vi "index.vi"() -> ()   [LabVIEW 2026]
uses:
  <vilib>/Utility/miscctls.llb/LVPoint32TypeDef.ctl
  <vilib>/Utility/miscctls.llb/LVRectTypeDef.ctl
  <vilib>/Utility/miscctls.llb/LVPointTypeDef.ctl
  <vilib>/Instr/_visa.llb/VISA Flush IO Buffer Mask.ctl
  <userlib>/Sensor.ctl
  <vilib>/measure/maspectr.llb/FFT Spectrum (Mag-Phase) for N Chan.vi
  <vilib>/Analysis/3filter.llb/Butterworth Filter (DBL).vi
  <vilib>/Instr/_visa.llb/VISA Configure Serial Port (Instr).vi
  <vilib>/measure/NI_MAPro.lvlib
  <vilib>/Analysis/NI_AALBase.lvlib
panel:
  out "AlphaxBeta":bool
  out "CoordsEEGBeta":T1 {"Čas (s)" format="%#.2f"; "Amplituda (mV)" format="%#.3f"}
  out "CoordsEEGAlpha":T1 {"Čas (s)" format="%#.2f"; "Amplituda (mV)" format="%#.3f"}
  out "SyncStopEEG":bool
  out "SyncStopACC":bool
  out "CoordsACC":T1 {"Čas (s)" format="%#.2f"; "Amplituda (mV)" format="%#.3f"}
  out "CoordsEMG":T1 {"Čas (s)" format="%#.2f"; "Amplituda (mV)" format="%#.3f"}
  out "EKGxHRV":bool
  out "CoordsHRV":T1 {"Čas (s)" format="%#.2f"; "Amplituda (mV)" format="%#.3f"}
  out "CoordsEKG":T1 {"Čas (s)" format="%#.2f"; "Amplituda (mV)" format="%#.3f"}
  out "GraphEEG2":waveform(dbl)(graph)
  out "GraphEEG1":waveform(dbl)(graph)
  out "error out 7":errorcluster
  out "error out 6":errorcluster
  out "RawEEG":waveform(dbl)(graph)
  out "size(s) 3":i32
  out "size(s) 4":i32
  out "error out 5":errorcluster
  out "error out 4":errorcluster
  out "Vzorkovacka 2":dbl
  out "RawACC":waveform(dbl)
  out "vzorkovackaEEG":dbl
  out "RawEMG":waveform(dbl)
  out "error out 3":errorcluster
  out "error out 2":errorcluster
  out "error out":errorcluster
  out "RawEKG":waveform(dbl)
  out "array":dbl[](array[numeric])
  out "Vzorkovacka":dbl
  out "SyncStopEMG":bool
  in  "Time Target (s)":dbl=60.0
  out "SyncStopEKG":bool
  in  "UvodniStranka":bool
  in  "ExitApp":bool
  in  "error in (no error)":errorcluster
  in  "Tab Control":T2(tab)
  in  "Playground":bool
  in  "UlohaACC":bool
  in  "UlohaEEG":bool
  in  "UlohaEMG":bool
  in  "UlohaEKG":bool
  out "EKGHRV":cluster{dbl[], dbl[]}(graph)
  in  "Délka časového okna (s)":dbl=1.0 min=1.0 max=20.0 step=1.0
  in  "Zobrazit graf č.":dbl min=0.0 max=0.0 step=1.0
  in  "DeleteSignalEKG":bool
  in  "StartMeasureEKG":bool
  in  "HintEKG":bool
  out "GraphEKG":waveform(dbl)[](graph)
  out "ChartEKG":dbl(graph)
  in  "Vstupní COM port 2":refnum<visa-resource-name>
  out "BPM":i32
  in  "Doba měření (s)":dbl=1.0 caption="Time Target (s)"
  in  "SaveCSV":bool
  in  "SavePNG":bool
  out "InfoCursor":cluster{"Čas (s)":dbl, "Amplituda (mV)":dbl}[](array[cluster]) {"Amplituda (mV)" format="%#.2f"; "Čas (s)" format="%#.2f"}
  in  "StopMeasureEKG":bool
  out "InfoCursorEEG":cluster{"Čas (s)":dbl, "Amplituda (mV)":dbl}[](array[cluster]) {"Amplituda (mV)" format="%#.2f"; "Čas (s)" format="%#.2f"}
  in  "Časové okno všech signálů (s)":dbl min=0.0 max=20.0 step=1.0
  in  "Zobrazit signál č._EEG":dbl min=0.0 max=1.0
  in  "HintEEG":bool
  in  "DeleteSignalEEG":bool
  in  "StartMeasureEEG":bool
  in  "Doba měření (s)":dbl
  in  "Vstupní COM port 4":refnum<visa-resource-name>
  out "GraphEEG4":waveform(dbl)(graph)
  out "GraphEEG3":waveform(dbl)(graph)
  out "ChartEEG":dbl(graph)
  in  "SaveCSVEEG":bool
  in  "StopMeasureEEG":bool
  out "InfoCursorACC":cluster{"Čas (s)":dbl, "Amplituda (mV)":dbl}[](array[cluster]) {"Amplituda (mV)" format="%#.2f"; "Čas (s)" format="%#.2f"}
  in  "SaveCSVACC":bool
  in  "SavePNGACC":bool
  in  "Délka časového okna (s) ACC":dbl=1.0 min=1.0 max=20.0 step=1.0
  in  "Zobrazit signál č._ACC":dbl min=0.0 max=1.0
  in  "HintACC":bool
  out "GraphACC":waveform(dbl)[](graph)
  out "ChartACC":dbl(graph)
  in  "DeleteSignalACC":bool
  in  "StartMeasureACC":bool
  in  "Doba měření (s) ACC":dbl
  in  "Vstupní COM port ACC":refnum<visa-resource-name>
  in  "StopMeasureACC":bool
  out "InfoCursorEMG":cluster{"Čas (s)":dbl, "Amplituda (mV)":dbl}[](array[cluster]) {"Amplituda (mV)" format="%#.2f"; "Čas (s)" format="%#.2f"}
  in  "SaveCSVEMG":bool
  in  "SavePNGEMG":bool
  in  "Délka časového okna (s) EMG":dbl=1.0 min=1.0 max=20.0 step=1.0
  in  "Zobrazit signál č.":dbl min=0.0 max=2.0
  in  "HintEMG":bool
  out "GraphEMG":waveform(dbl)[](graph)
  out "ChartEMG":dbl(graph)
  in  "DeleteSignalEMG":bool
  in  "StartMeasureEMG":bool
  in  "Doba měření (s)":dbl
  in  "Vstupní COM port 3":refnum<visa-resource-name>
  in  "StopMeasureEMG":bool
  out "SpectrumPlayground":cluster{"f0":dbl, "df":dbl, "magnitude":dbl[]}[](graph)
  in  "Filtr":bool
  in  "SaveFileButton":bool
  out "Waveform Graph":waveform(dbl)[](graph)
  in  "Horní mezní frekvence":dbl=0.45000000000000007 format="%0.2f"
  in  "Dolní mezní frekvence":dbl=0.12500000000000006 format="%0.4f"
  in  "Typ filtru":T3(ring)
  in  "OdstranitFiltr":bool
  in  "Cluster":T4
  in  "DeleteSignal":bool
  out "Waveform Chart":dbl[](graph)
  in  "SendToFilter":bool
  out "Waveform":waveform(dbl)[](graph)
  out "SyncStop":bool
  in  "Vstupní COM port":refnum<visa-resource-name>
  in  "Vzorkovací frekvence (Hz)":enum16{"1", "10", "100", "1000"}(ring)
  in  "Druh signálu":T5
  in  "StartMeasure":bool
  in  "StopMeasure":bool
  in  "index":i32
  # "CHYBÍ UDĚLAT SMARTKURSOR A STOP BUTTON U EEG\nUDĚLAT VŠECHNY PROTOKOLY\nUDĚLAT PEAK COUNTER V AKCELEROMETRU\nFIXNOUT VOLNÉ MĚŘENÍ"
  # "Aplikace pro měření na platformě PLUX BITalino"
  # "Úloha č. 1 - měření a vyhodnocení EKG signálu"
  # "Vstupní COM port"
  # "Kurzor"
  # "Amplituda (mV) / BPM (-)"
  # "Čas (s)"
  # "Úloha č. 3 - měření a vyhodnocení EEG signálu"
  # "Vstupní COM port"
  # "Zobrazit graf č."
  # "Alfa"
  # "Beta"
  # "Kurzor"
  # "Amplituda (uV)"
  # "Čas (s)"
  # "EDA"
  # "Úloha č. 4 - měření a vyhodnocení signálu Z - akcelerometru"
  # "Vstupní COM port"
  # "Doba měření (s)"
  # "Zobrazit signál č."
  # "Délka časového okna (s)"
  # "Kurzor"
  # "Amplituda (g)"
  # "Čas (s)"
  # "Úloha č. 2 - měření a vyhodnocení EMG signálu"
  # "Vstupní COM port"
  # "Délka časového okna (s)"
  # "Kurzor"
  # "Amplituda (mV)"
  # "Čas (s)"
  # "A1"
  # "A2"
  # "A3"
  # "A4"
  # "A5"
  # "A6"
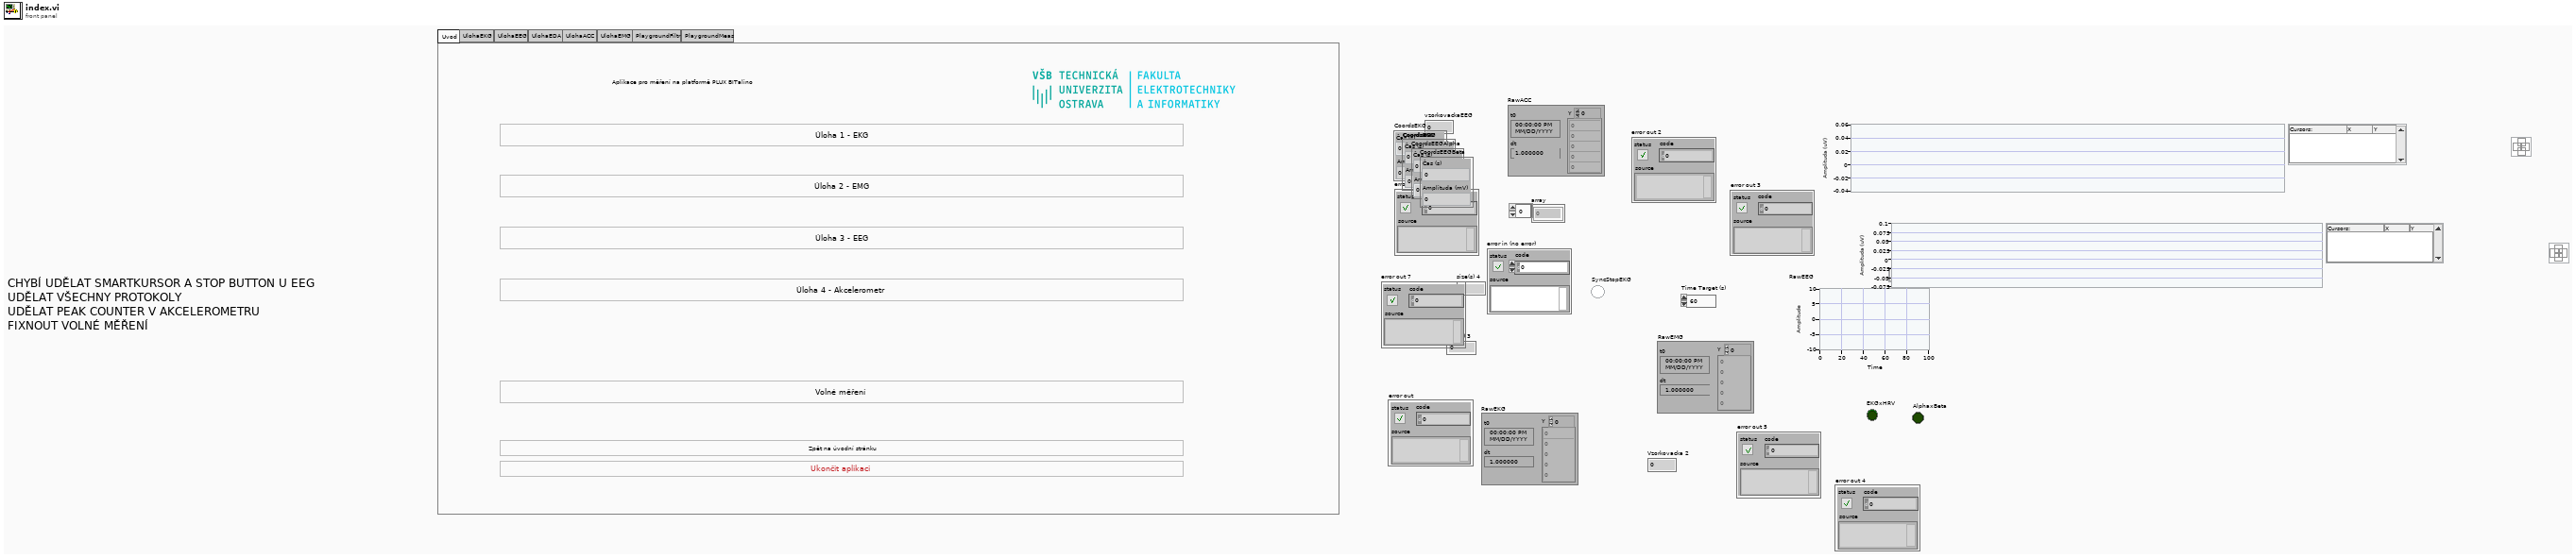
[diagram p1: front panel]
types:
  T1 = typedef "LVPoint32TypeDef.ctl" = cluster{"Čas (s)":dbl, "Amplituda (mV)":dbl}
  T2 = enum32{"Uvod", "UlohaEKG", "UlohaEEG", "UlohaEDA", "UlohaACC", "UlohaEMG", "PlaygroundFiltr", "PlaygroundMeas"}
  T3 = enum32{"Lowpass", "Highpass", "Bandpass", "Bandstop"}
  T4 = cluster{"A1":bool, "A2":bool, "A3":bool, "A4":bool, "A5":bool, "A6":bool}
  T5 = cluster{"Signál na kanálu A1":enum16{"EMG", "ECG", "EEG", "EDA", "ACC"}, "Signál na kanálu A2":enum16{"EMG", "ECG", "EEG", "EDA", "ACC"}, "Signál na kanálu A3":enum16{"EMG", "ECG", "EEG", "EDA", "ACC"}, "Signál na kanálu A4":enum16{"EMG", "ECG", "EEG", "EDA", "ACC"}, "Signál na kanálu A5":enum16{"EMG", "ECG", "EEG", "EDA", "ACC"}, "Signál na kanálu A6":enum16{"EMG", "ECG", "EEG", "EDA", "ACC"}}
  T6 = enum16{"Always On", "Always Off", "Off While Running"}
  T7 = enum16{"Wait", "Exit", "Measure", "Intro", "UlohaEKG", "UlohaEMG", "PlaygroundMeas", "UlohaEEG", "UlohaEDA", "UlohaACC", "PlaygroundFiltr", "SaveFile", "FilterSignal", "RemoveFilter", "HintEKG", "DeleteSignal", "DeleteSignalEKG", "HintEMG", "HintEEG", "DeleteSignalEMG", "StartMeasureEEG", "DeleteSignalEEG", "ShowGraphECG", "ChangeTimeECG", "SavePNG", "SaveCSV", "ChangeTimeEMG", "ShowGraphEMG", "ShowGraphEEG", "ShowGraphACC", "ChangeTimeACC", "DeleteSignalACC", "HintACC", "ChangeTimeEEG", "Cursor"}
  T8 = enum32{"Uvod", "UlohaEKG", "UlohaEEG", "UlohaEDA", "UlohaACC", "UlohaEMG", "PlaygroundFiltr"}
  T9 = typedef "LVPointTypeDef.ctl" = cluster{"Horizontal":i16, "Vertical":i16}
  T10 = typedef "LVRectTypeDef.ctl" = cluster{"Left":i16, "Top":i16, "Right":i16, "Bottom":i16}
  T11 = enum8{"Enabled", "Disabled", "Disabled and Grayed Out"}
  T12 = typedef "Sensor.ctl" = enum16{"EMG", "ECG", "EEG", "EDA", "ACC", "LUX"}
  T13 = cluster{"Sensor 1":T12, "Sensor 2":T12, "Sensor 3":T12, "Sensor 4":T12, "Sensor 5":T12, "Sensor 6":T12}
  T14 = typedef "VISA Flush IO Buffer Mask.ctl" = u16
  T15 = cluster{"Result":dbl, "Result":dbl, "Result":dbl, "Result":dbl, "Result":dbl, "Result":dbl}
  T16 = enum16{"Wait", "Exit", "Measure", "Intro", "UlohaEKG", "UlohaEMG", "PlaygroundMeas", "UlohaEEG", "UlohaEDA", "UlohaACC", "PlaygroundFiltr", "SaveFile", "FilterSignal", "RemoveFilter", "HintEKG"}
  T17 = enum16{"Wait", "Exit", "Measure", "Intro", "UlohaEKG", "UlohaEMG", "PlaygroundMeas", "UlohaEEG", "UlohaEDA", "UlohaACC"}
  T18 = enum16{"Wait", "Exit", "Measure", "Intro", "UlohaEKG", "UlohaEMG", "PlaygroundMeas"}
  T19 = enum16{"Wait", "Exit", "Measure", "Intro", "UlohaEKG", "UlohaEMG"}
  T20 = enum16{"Wait", "Exit", "Measure", "Intro", "UlohaEKG", "UlohaEMG", "PlaygroundMeas", "UlohaEEG", "UlohaEDA", "UlohaACC", "PlaygroundFiltr", "SaveFile", "FilterSignal", "RemoveFilter", "HintEKG", "DeleteSignal", "DeleteSignalEKG", "HintEMG", "HintEEG", "DeleteSignalEMG", "StartMeasureEEG", "DeleteSignalEEG", "ShowGraphECG", "ChangeTimeECG", "SavePNG", "SaveCSV", "ChangeTimeEMG", "ShowGraphEMG", "ShowGraphEEG", "ShowGraphACC", "ChangeTimeACC", "DeleteSignalACC"}
  T21 = enum16{"Wait", "Exit", "Measure", "Intro", "UlohaEKG", "UlohaEMG", "PlaygroundMeas", "UlohaEEG", "UlohaEDA", "UlohaACC", "PlaygroundFiltr", "SaveFile", "FilterSignal", "RemoveFilter", "HintEKG", "DeleteSignal"}
  T22 = enum16{"Wait", "Exit", "Measure", "Intro", "UlohaEKG", "UlohaEMG", "PlaygroundMeas", "UlohaEEG", "UlohaEDA", "UlohaACC", "PlaygroundFiltr", "SaveFile", "FilterSignal", "RemoveFilter", "HintEKG", "DeleteSignal", "DeleteSignalEKG"}
  T23 = enum16{"Wait", "Exit", "Measure", "Intro", "UlohaEKG", "UlohaEMG", "PlaygroundMeas", "UlohaEEG", "UlohaEDA", "UlohaACC", "PlaygroundFiltr", "SaveFile", "FilterSignal", "RemoveFilter", "HintEKG", "DeleteSignal", "DeleteSignalEKG", "HintEMG", "HintEEG", "DeleteSignalEMG"}
  T24 = enum16{"Wait", "Exit", "Measure", "Intro", "UlohaEKG", "UlohaEMG", "PlaygroundMeas", "UlohaEEG", "UlohaEDA", "UlohaACC", "PlaygroundFiltr", "SaveFile", "FilterSignal", "RemoveFilter", "HintEKG", "DeleteSignal", "DeleteSignalEKG", "HintEMG", "HintEEG", "DeleteSignalEMG", "StartMeasureEEG", "DeleteSignalEEG"}
  T25 = enum16{"Wait", "Exit", "Measure", "Intro", "UlohaEKG", "UlohaEMG", "PlaygroundMeas", "UlohaEEG", "UlohaEDA", "UlohaACC", "PlaygroundFiltr", "SaveFile", "FilterSignal", "RemoveFilter", "HintEKG", "DeleteSignal", "DeleteSignalEKG", "HintEMG", "HintEEG", "DeleteSignalEMG", "StartMeasureEEG", "DeleteSignalEEG", "ShowGraphECG", "ChangeTimeECG"}
  T26 = enum16{"Wait", "Exit", "Measure", "Intro", "UlohaEKG", "UlohaEMG", "PlaygroundMeas", "UlohaEEG", "UlohaEDA", "UlohaACC", "PlaygroundFiltr", "SaveFile", "FilterSignal", "RemoveFilter", "HintEKG", "DeleteSignal", "DeleteSignalEKG", "HintEMG", "HintEEG", "DeleteSignalEMG", "StartMeasureEEG", "DeleteSignalEEG", "ShowGraphECG", "ChangeTimeECG", "SavePNG", "SaveCSV", "ChangeTimeEMG"}
  T27 = enum16{"Wait", "Exit", "Measure", "Intro", "UlohaEKG", "UlohaEMG", "PlaygroundMeas", "UlohaEEG", "UlohaEDA", "UlohaACC", "PlaygroundFiltr", "SaveFile", "FilterSignal", "RemoveFilter", "HintEKG", "DeleteSignal", "DeleteSignalEKG", "HintEMG", "HintEEG", "DeleteSignalEMG", "StartMeasureEEG", "DeleteSignalEEG", "ShowGraphECG", "ChangeTimeECG", "SavePNG", "SaveCSV", "ChangeTimeEMG", "ShowGraphEMG", "ShowGraphEEG", "ShowGraphACC", "ChangeTimeACC", "DeleteSignalACC", "HintACC", "ChangeTimeEEG"}
  T28 = enum16{"Wait", "Exit", "Measure", "Intro", "UlohaEKG", "UlohaEMG", "PlaygroundMeas", "UlohaEEG", "UlohaEDA", "UlohaACC", "PlaygroundFiltr", "SaveFile", "FilterSignal", "RemoveFilter", "HintEKG", "DeleteSignal", "DeleteSignalEKG", "HintEMG", "HintEEG", "DeleteSignalEMG", "StartMeasureEEG", "DeleteSignalEEG", "ShowGraphECG", "ChangeTimeECG", "SavePNG"}
  T29 = enum16{"Wait", "Exit", "Measure", "Intro", "UlohaEKG", "UlohaEMG", "PlaygroundMeas", "UlohaEEG", "UlohaEDA", "UlohaACC", "PlaygroundFiltr", "SaveFile", "FilterSignal", "RemoveFilter", "HintEKG", "DeleteSignal", "DeleteSignalEKG", "HintEMG", "HintEEG", "DeleteSignalEMG", "StartMeasureEEG", "DeleteSignalEEG", "ShowGraphECG", "ChangeTimeECG", "SavePNG", "SaveCSV"}
  T30 = enum16{"Wait", "Exit", "Measure", "Intro", "UlohaEKG", "UlohaEMG", "PlaygroundMeas", "UlohaEEG", "UlohaEDA", "UlohaACC", "PlaygroundFiltr", "SaveFile", "FilterSignal", "RemoveFilter", "HintEKG", "DeleteSignal", "DeleteSignalEKG", "HintEMG", "HintEEG", "DeleteSignalEMG", "StartMeasureEEG", "DeleteSignalEEG", "ShowGraphECG", "ChangeTimeECG", "SavePNG", "SaveCSV", "ChangeTimeEMG", "ShowGraphEMG", "ShowGraphEEG"}
  T31 = enum16{"Wait", "Exit", "Measure", "Intro", "UlohaEKG", "UlohaEMG", "PlaygroundMeas", "UlohaEEG", "UlohaEDA", "UlohaACC", "PlaygroundFiltr", "SaveFile", "FilterSignal", "RemoveFilter", "HintEKG", "DeleteSignal", "DeleteSignalEKG", "HintEMG", "HintEEG", "DeleteSignalEMG", "StartMeasureEEG", "DeleteSignalEEG", "ShowGraphECG", "ChangeTimeECG", "SavePNG", "SaveCSV", "ChangeTimeEMG", "ShowGraphEMG"}
  T32 = enum16{"Wait", "Exit", "Measure", "Intro", "UlohaEKG", "UlohaEMG", "PlaygroundMeas", "UlohaEEG", "UlohaEDA", "UlohaACC", "PlaygroundFiltr", "SaveFile", "FilterSignal", "RemoveFilter", "HintEKG", "DeleteSignal", "DeleteSignalEKG", "HintEMG", "HintEEG", "DeleteSignalEMG", "StartMeasureEEG", "DeleteSignalEEG", "ShowGraphECG", "ChangeTimeECG", "SavePNG", "SaveCSV", "ChangeTimeEMG", "ShowGraphEMG", "ShowGraphEEG", "ShowGraphACC", "ChangeTimeACC", "DeleteSignalACC", "HintACC"}
  T33 = enum16{"Wait", "Exit", "Measure", "Intro", "UlohaEKG", "UlohaEMG", "PlaygroundMeas", "UlohaEEG", "UlohaEDA", "UlohaACC", "PlaygroundFiltr", "SaveFile", "FilterSignal", "RemoveFilter", "HintEKG", "DeleteSignal", "DeleteSignalEKG", "HintEMG", "HintEEG", "DeleteSignalEMG", "StartMeasureEEG", "DeleteSignalEEG", "ShowGraphECG"}
  T34 = enum16{"Wait", "Exit", "Measure", "Intro", "UlohaEKG", "UlohaEMG", "PlaygroundMeas", "UlohaEEG", "UlohaEDA", "UlohaACC", "PlaygroundFiltr"}
  T35 = enum16{"Wait", "Exit", "Measure", "Intro", "UlohaEKG", "UlohaEMG", "PlaygroundMeas", "UlohaEEG", "UlohaEDA", "UlohaACC", "PlaygroundFiltr", "SaveFile"}
  T36 = enum16{"Wait", "Exit", "Measure", "Intro", "UlohaEKG", "UlohaEMG", "PlaygroundMeas", "UlohaEEG", "UlohaEDA", "UlohaACC", "PlaygroundFiltr", "SaveFile", "FilterSignal", "RemoveFilter"}
  T37 = enum16{"Wait", "Exit", "Measure", "Intro", "UlohaEKG", "UlohaEMG", "PlaygroundMeas", "UlohaEEG", "UlohaEDA", "UlohaACC", "PlaygroundFiltr", "SaveFile", "FilterSignal", "RemoveFilter", "HintEKG", "DeleteSignal", "DeleteSignalEKG", "HintEMG"}
  T38 = enum16{"Wait", "Exit", "Measure", "Intro", "UlohaEKG", "UlohaEMG", "PlaygroundMeas", "UlohaEEG", "UlohaEDA", "UlohaACC", "PlaygroundFiltr", "SaveFile", "FilterSignal", "RemoveFilter", "HintEKG", "DeleteSignal", "DeleteSignalEKG", "HintEMG", "HintEEG"}
  T39 = typedef "LVRangeTypeDef.ctl" = cluster{"Minimum":dbl, "Maximum":dbl, "Increment":dbl, "Minor Increment":dbl, "Start":dbl}
  T40 = typedef "LVPoint32TypeDef.ctl" = cluster{"Horizontal":i32, "Vertical":i32}
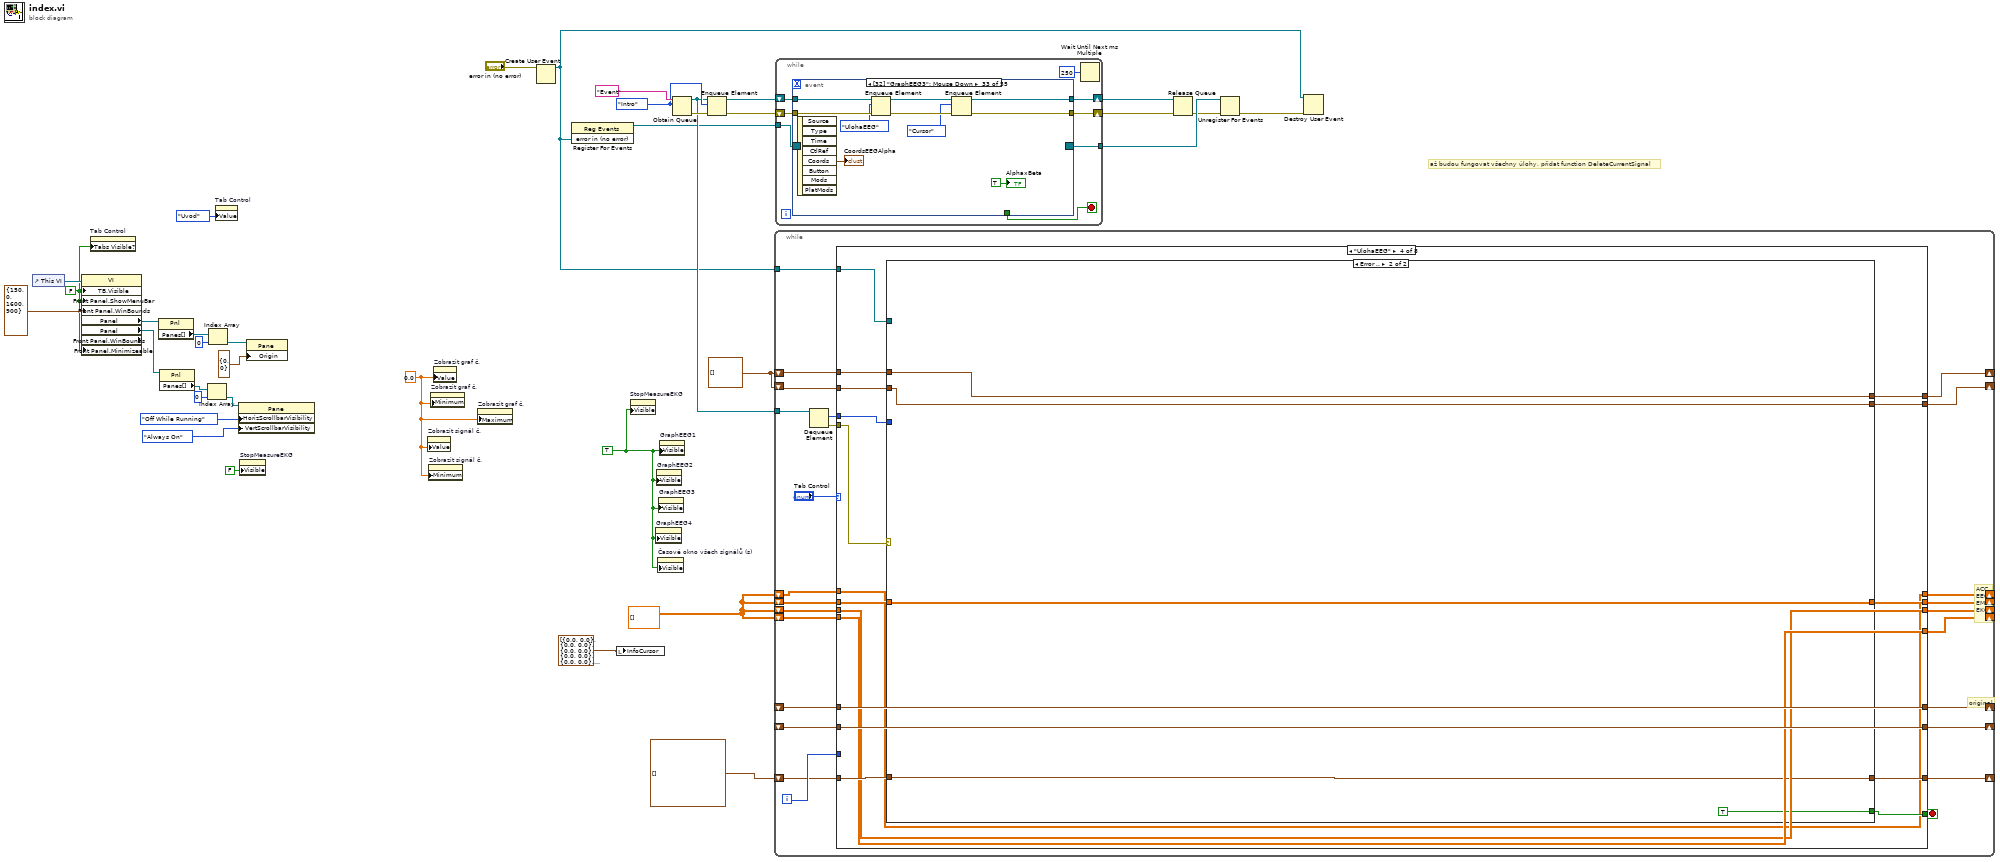
[diagram p0: block diagram]
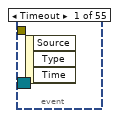
[diagram p2: hidden frame]
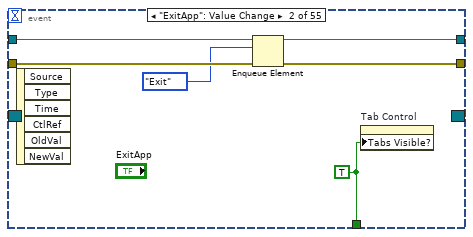
[diagram p3: hidden frame]
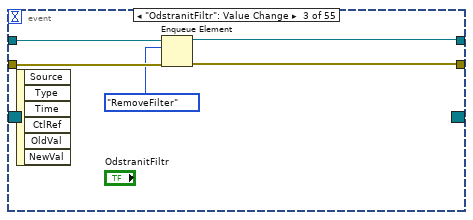
[diagram p4: hidden frame]
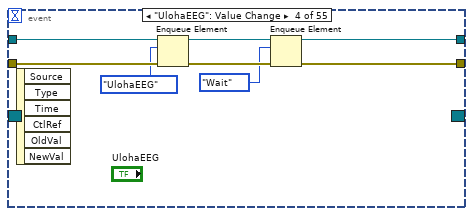
[diagram p5: hidden frame]
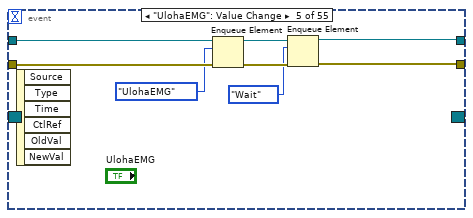
[diagram p6: hidden frame]
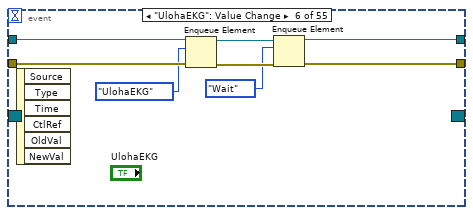
[diagram p7: hidden frame]
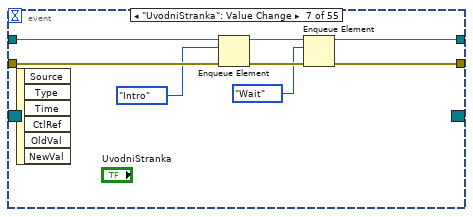
[diagram p8: hidden frame]
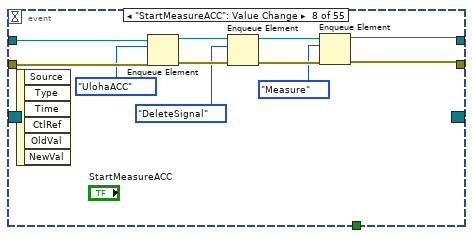
[diagram p9: hidden frame]
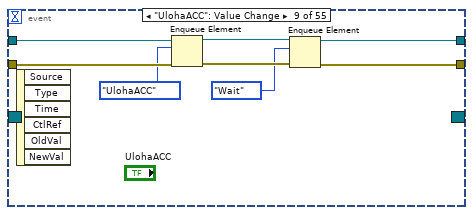
[diagram p10: hidden frame]
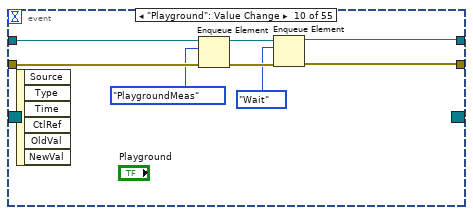
[diagram p11: hidden frame]
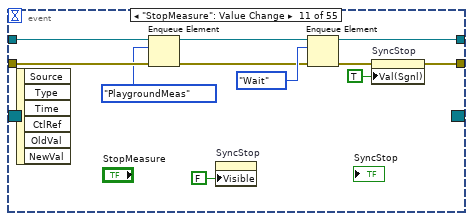
[diagram p12: hidden frame]
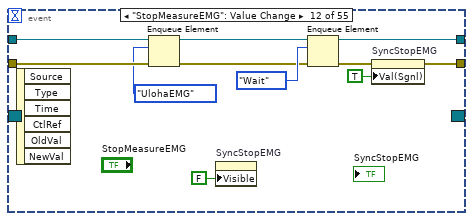
[diagram p13: hidden frame]
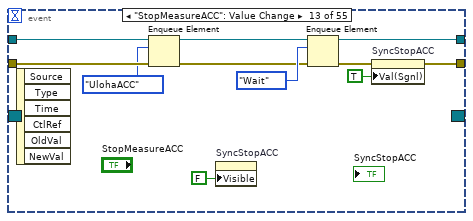
[diagram p14: hidden frame]
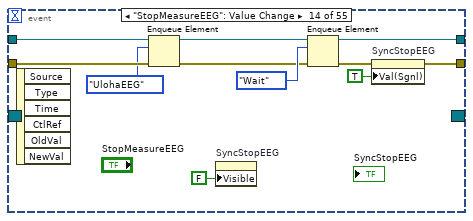
[diagram p15: hidden frame]
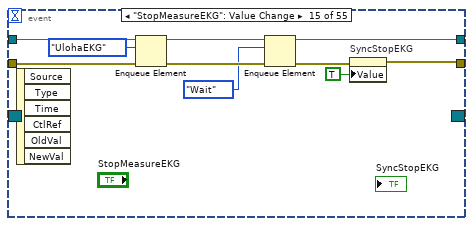
[diagram p16: hidden frame]
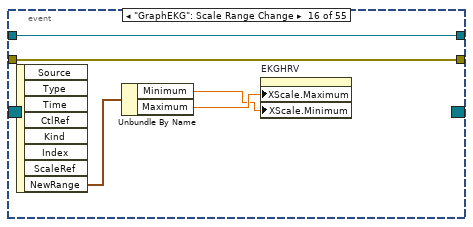
[diagram p17: hidden frame]
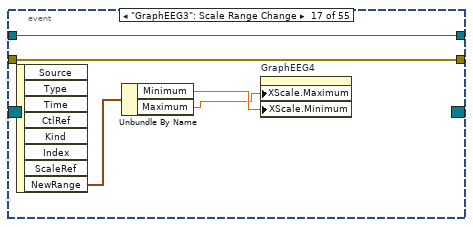
[diagram p18: hidden frame]
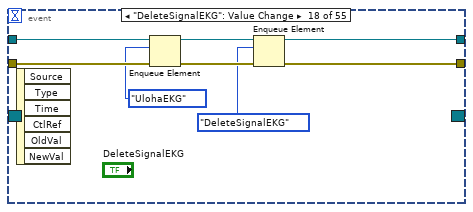
[diagram p19: hidden frame]
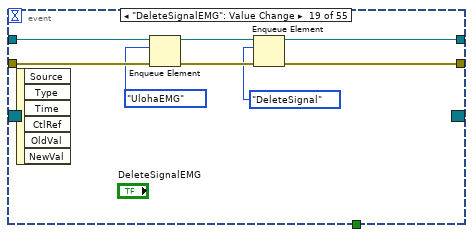
[diagram p20: hidden frame]
diagram:
  w2 = cluster{"X":dbl, "Y":dbl}[] []
  w3 = TRUE
  w5 = 0.0 ("Zobrazit graf č.")
  w4 = dbl[][] []
  w18 = T7."Intro"
  w23 = FALSE ("Front Panel Window:Closeable")
  # "až budou fungovat všechny úlohy, přidat function DeleteCurrentSignal"
  # "ACC\nEEG\nEMG\nEKG"
  # "original"
  n1 = control-ref of="This VI"() -> (w36:refnum<vi>)
  n2 = property class="VI" props=["TB.Visible", "Front Panel.ShowMenuBar", "Front Panel.WinBounds", "Panel", "Panel", "Front Panel.WinBounds", "Front Panel.Minimizeable"](reference=w36, "TB.Visible"=w23, "Front Panel.ShowMenuBar"=w23, "Front Panel.WinBounds"=T10 {"Left"=150, "Top"=0, "Right"=1600, "Bottom"=900} ("Front Panel Window:Window Bounds"), "Front Panel.Minimizeable"=w23) -> ("Panel"=w34:refnum<vi>, "Panel"=w28:refnum<vi>)  [unwired: 1 in, 3 out]
  n3 = property on="Tab Control" class="TabCtl (strict)"("Tabs Visible?"=w23) -> ()  [unwired: 2 in, 2 out]
  n4 = property class="Pnl"(reference=w34) -> ("Panes[]"=w33:refnum<vi>[])  [unwired: 1 in, 2 out]
  n5 = property class="Pnl"(reference=w28) -> ("Panes[]"=w27:refnum<vi>[])  [unwired: 1 in, 2 out]
  n6 = Index Array(array=w27, index=0) -> (element=w25:refnum<vi>)
  n7 = Index Array(array=w33, index=0) -> (element=w31:refnum<vi>)
  n8 = property on="Tab Control" class="TabCtl (strict)"("Value"=T8."Uvod" ("Tab Control")) -> ()  [unwired: 2 in, 2 out]
  n9 = property class="Pane"(reference=w25, "HorizScrollbarVisibility"=T6."Off While Running" ("Horizontal Scrollbar Visibility"), "VertScrollbarVisibility"=T6."Always On" ("Vertical Scrollbar Visibility")) -> ()  [unwired: 1 in, 2 out]
  n10 = property on="StopMeasureEKG" class="Bool (strict)"("Visible"=FALSE) -> ()  [unwired: 2 in, 2 out]
  n11 = property class="Pane"(reference=w31, "Origin"=T9 {"Horizontal"=0, "Vertical"=0}) -> ()  [unwired: 1 in, 2 out]
  n12 = property on="Zobrazit signál č." class="DigNum (strict)"("Value"=w5) -> ()  [unwired: 2 in, 2 out]
  n13 = property on="Zobrazit signál č." class="DigNum (strict)"("Minimum"=w5) -> ()  [unwired: 2 in, 2 out]
  n14 = property on="Zobrazit graf č." class="DigNum (strict)"("Minimum"=w5) -> ()  [unwired: 2 in, 2 out]
  n15 = property on="Zobrazit graf č." class="DigNum (strict)"("Value"=w5) -> ()  [unwired: 2 in, 2 out]
  n16 = property on="Zobrazit graf č." class="DigNum (strict)"("Maximum"=w5) -> ()  [unwired: 2 in, 2 out]
  n17 = Create User Event(user event datatype="error in (no error)") -> (user event=w10:refnum<user-event>)  [unwired: 1 in, 1 out]
  n18 = register-events(w10) -> (reference out=w9:refnum<event-registration>)  [unwired: 2 in, 1 out]
  n19 = local write "InfoCursor"(cluster{dbl, dbl}[] [{0.0, 0.0}, {0.0, 0.0}, {0.0, 0.0}, {0.0, 0.0}, {0.0, 0.0}, {0.0, 0.0}, {0.0, 0.0}, {0.0, 0.0}, {0.0, 0.0}, {0.0, 0.0}, {0.0, 0.0}, {0.0, 0.0}, {0.0, 0.0}, {0.0, 0.0}, {0.0, 0.0}, {0.0, 0.0}, {0.0, 0.0}, {0.0, 0.0}, {0.0, 0.0}, {0.0, 0.0}, {0.0, 0.0}, {0.0, 0.0}] ("InfoCursor")) -> ()
  n20 = property on="StopMeasureEKG" class="Bool (strict)"("Visible"=w3) -> ()  [unwired: 2 in, 2 out]
  n21 = property on="GraphEEG4" class="WFGraph (strict)"("Visible"=w3) -> ()  [unwired: 2 in, 2 out]
  n22 = property on="GraphEEG2" class="WFGraph (strict)"("Visible"=w3) -> ()  [unwired: 2 in, 2 out]
  n23 = property on="Časové okno všech signálů (s)" class="DigNum (strict)"("Visible"=w3) -> ()  [unwired: 2 in, 2 out]
  n24 = property on="GraphEEG3" class="WFGraph (strict)"("Visible"=w3) -> ()  [unwired: 2 in, 2 out]
  n25 = property on="GraphEEG1" class="WFGraph (strict)"("Visible"=w3) -> ()  [unwired: 2 in, 2 out]
  n26 = Obtain Queue(name (unnamed)="Event", element data type=w18) -> (queue out=w17:refnum<queue>, error out=w21:errorcluster)  [unwired: 3 in, 1 out]
  n27 = Enqueue Element(queue=w17, element=w18, error in (no error)=w21) -> (queue out=w20:refnum<queue>, error out=w19:errorcluster)  [unwired: 1 in, 1 out]
  n28 = while {
    shift-right: [w61] -> _
    shift-left: _ -> [w54]
    tunnel: w17 -> [w57]
    tunnel: w10 -> [w56]
    shift-right: [w53] -> _
    shift-left: _ -> [w52]
    shift-right: [w51] -> _
    shift-left: waveform(dbl)[] [] -> [w50]
    shift-right: [w45] -> _
    shift-left: w4 -> [w48]
    shift-right: [w46] -> _
    shift-left: w4 -> [w47]
    shift-right: [w43] -> _
    shift-left: w4 -> [w44]
    shift-right: [w41] -> _
    shift-left: w4 -> [w42]
    shift-right: [w39] -> _
    shift-left: w2 -> [w40]
    shift-right: [w37] -> _
    shift-left: w2 -> [w38]
    i -> [w60]
    stop <- w49 stop-if-true
    n29 = Dequeue Element(queue=w57) -> (element=w58:T7, error out=w55:errorcluster)  [unwired: 2 in, 2 out]
    n30 = case shown="\"UlohaEEG\"" "Tab Control" {
      tunnel: [w72 w94 w139 w340 w531 w551 w713 w874] -> w61
      tunnel: w54 -> [w72 w95 w139 w340 w531 w551 w713 w871]
      tunnel: w60 -> [_ _ _ _ _ _ _ _]
      tunnel: w58 -> [w71 w96 w142 w339 w530 w544 w712 w880]
      tunnel: w56 -> [_ _ w141 w335 _ w545 w708 w879]
      tunnel: w55 -> [_ _ w136 w334 _ w543 w707 w878]
      tunnel: [w70 w93 w140 w338 w529 w550 w711 w877] -> w53
      tunnel: w52 -> [w70 w92 w140 w338 w529 w550 w711 w877]
      tunnel: [w69 w91 w138 w337 w528 w539 w709 w876] -> w51
      tunnel: w50 -> [w69 w91 w137 w336 w528 w540 w710 w876]
      tunnel: [FALSE FALSE w135 w333 FALSE FALSE w706 w875] -> w49
      tunnel: [w67 w89 w134 w332 w526 w548 w703 w873] -> w45
      tunnel: w48 -> [w67 w89 w133 w332 w526 w548 w703 w873]
      tunnel: w47 -> [w66 w88 w132 w331 w525 w547 w705 w872]
      tunnel: [w66 w88 w132 w331 w525 w547 w704 w872] -> w46
      tunnel: w44 -> [w65 w87 w131 w330 w524 w546 w702 w870]
      tunnel: [w65 w87 w131 w329 w524 w546 w702 w870] -> w43
      tunnel: w42 -> [w64 w86 w130 w328 w523 w542 w701 w869]
      tunnel: [w64 w86 w130 w328 w523 w541 w701 w869] -> w41
      tunnel: w40 -> [w63 w85 w129 w327 w522 w538 w700 w868]
      tunnel: [w63 w85 w128 w326 w522 w538 w700 w868] -> w39
      tunnel: w38 -> [w62 w84 w127 w325 w521 w537 w699 w867]
      tunnel: [w62 w84 w126 w324 w521 w536 w698 w867] -> w37
      frame "Uvod", Default {
        n31 = case shown="\"UlohaEKG\"" w71 {
          frame "Wait", Default {
            n32 = property on="UvodniStranka" class="Bool"("DisabledEnum"=T11."Disabled and Grayed Out" ("Disabled")) -> ()  [unwired: 2 in, 2 out]
            n33 = property on="Tab Control" class="TabCtl (strict)"("Tabs Visible?"=FALSE) -> ()  [unwired: 2 in, 2 out]
          }
          frame "UlohaEKG" {
            n34 = property on="Tab Control" class="TabCtl (strict)"("Value"=T2."UlohaEKG" ("Tab Control")) -> ()  [unwired: 2 in, 2 out]
          }
          frame "UlohaEMG" {
            n35 = property on="Tab Control" class="TabCtl (strict)"("Value"=T2."UlohaEMG" ("Tab Control")) -> ()  [unwired: 2 in, 2 out]
          }
          frame "Exit" {
            n36 = flat-sequence {
              frame #0 {
                n37 = property on="Tab Control" class="TabCtl (strict)"("Value"=T2."Uvod" ("Tab Control")) -> ()  [unwired: 2 in, 2 out]
              }
              frame #1 {
                n38 = Stop(stop? (T)=TRUE) -> ()
              }
            }
          }
          frame "Intro" {
            n39 = property on="Tab Control" class="TabCtl (strict)"("Value"=T2."Uvod" ("Tab Control")) -> ()  [unwired: 2 in, 2 out]
          }
          frame "PlaygroundMeas" {
            n40 = property on="Tab Control" class="TabCtl (strict)"("Value"=T2."PlaygroundMeas" ("Tab Control")) -> ()  [unwired: 2 in, 2 out]
          }
          frame "Measure" {
          }
          frame "UlohaEEG" {
            n41 = property on="Tab Control" class="TabCtl (strict)"("Value"=T2."UlohaEEG" ("Tab Control")) -> ()  [unwired: 2 in, 2 out]
          }
          frame "UlohaEDA" {
            n42 = property on="Tab Control" class="TabCtl (strict)"("Value"=T2."UlohaEDA" ("Tab Control")) -> ()  [unwired: 2 in, 2 out]
          }
          frame "UlohaACC" {
            n43 = property on="Tab Control" class="TabCtl (strict)"("Value"=T2."UlohaACC" ("Tab Control")) -> ()  [unwired: 2 in, 2 out]
          }
          frame "PlaygroundFiltr" {
          }
        }
      }
      frame "PlaygroundFiltr" {
        n44 = case shown="\"Wait\", Default" w96 {
          tunnel: w95 -> [w97 w103 w116 w118 w122 w125]
          tunnel: [w97 w100 w116 w118 w122 w125] -> w94
          tunnel: [w97 w100 w114 w117 w121 w124] -> w93
          tunnel: w92 -> [_ w104 w114 w117 w121 w124]
          frame "Wait", Default {
            n45 = property on="UvodniStranka" class="Bool"("DisabledEnum"=T11."Enabled" ("Disabled")) -> ()  [unwired: 2 in, 2 out]
            n46 = call-poly <vilib>:"FFT Spectrum (Mag-Phase).vi"("time signals"=w97) -> ("magnitudes"=w98:cluster{"f0":dbl, "df":dbl, "magnitude":dbl[]}[])  [unwired: 6 in, 4 out]
            n47 = local write "SpectrumPlayground"(w98) -> ()
            "Waveform Graph" <- w97
          }
          frame "FilterSignal" {
            n48 = Index Array(array=w103, index="index") -> (element=w101:waveform(dbl))
            n49 = Unbundle By Name(w101) -> ("Y"=w108:dbl[], "dt"=w106:dbl)
            n50 = Reciprocal(x=w106) -> (1/x=w107:dbl)
            n51 = call-poly <vilib>:"Butterworth Filter.vi"("filter type"="Typ filtru", "low cutoff freq: fl"="Dolní mezní frekvence", "high cutoff freq: fh"="Horní mezní frekvence", "sampling freq: fs"=w107, "X"=w108) -> ("Filtered X"=w109:dbl[])  [unwired: 3 in, 1 out]
            n52 = Bundle By Name("Y"=w109, "dt"=w106) -> (w105:waveform(dbl))  [unwired: 1 in]
            n53 = Build Array (concatenate)(w104, w105) -> (w100:waveform(dbl)[])
            n54 = call-poly <vilib>:"FFT Spectrum (Mag-Phase).vi"("time signals"=w100) -> ("magnitudes"=→"SpectrumPlayground":cluster{"f0":dbl, "df":dbl, "magnitude":dbl[]}[])  [unwired: 6 in, 4 out]
            n55 = local write "Waveform Graph"(w100) -> ()
          }
          frame "RemoveFilter" {
            n56 = call-poly <vilib>:"FFT Spectrum (Mag-Phase).vi"("time signals"=w114) -> ("magnitudes"=w115:cluster{"f0":dbl, "df":dbl, "magnitude":dbl[]}[])  [unwired: 6 in, 4 out]
            n57 = local write "Waveform Graph"(w114) -> ()
            n58 = local write "SpectrumPlayground"(w115) -> ()
          }
          frame "Exit" {
            n59 = flat-sequence {
              frame #0 {
                n60 = property on="Tab Control" class="TabCtl (strict)"("Value"=T2."Uvod" ("Tab Control")) -> ()  [unwired: 2 in, 2 out]
              }
              frame #1 {
                n61 = Stop(stop? (T)=TRUE) -> ()
              }
            }
          }
          frame "Intro" {
            n62 = property on="Tab Control" class="TabCtl (strict)"("Value"=T2."Uvod" ("Tab Control")) -> ()  [unwired: 2 in, 2 out]
          }
          frame "SaveFile" {
          }
        }
      }
      frame "UlohaEKG" {
        n63 = case shown="No Error" w136 {
          tunnel: w142 -> [w153 _]
          tunnel: w141 -> [w152 _]
          tunnel: [w151 w323] -> w138
          tunnel: w137 -> [w150 w323]
          tunnel: [FALSE TRUE] -> w135
          tunnel: [w148 w321] -> w134
          tunnel: w133 -> [w147 w321]
          tunnel: w129 -> [w146 w320]
          tunnel: [w145 w320] -> w128
          tunnel: w127 -> [w144 w319]
          tunnel: [w143 w319] -> w126
          frame No Error {
            n64 = case shown="\"Cursor\"" w153 {
              tunnel: w152 -> [_ _ _ w218 _ _ _ _ _ _ _]
              tunnel: [w159 w168 w173 w188 w267 w279 w286 w291 w307 w313 w317] -> w151
              tunnel: w150 -> [w159 w168 w173 w187 w267 w279 w286 w291 _ w313 w317]
              tunnel: [w157 w169 w172 w183 w268 w280 w287 w293 w306 w312 w316] -> w148
              tunnel: w147 -> [w157 w169 w172 w185 w268 w280 w287 w293 w306 w312 w316]
              tunnel: w146 -> [w156 w165 w171 w179 w269 w277 w284 w290 w305 w311 w315]
              tunnel: [w156 w165 w171 w179 w259 w277 w284 w290 w305 w311 w315] -> w145
              tunnel: w144 -> [w155 w161 w170 w177 w262 w276 w283 w289 w304 w310 w314]
              tunnel: [w155 w161 w170 w177 w260 w276 w283 w289 w304 w310 w314] -> w143
              frame "Wait", Default {
                w154 = T11."Enabled" ("Disabled")
                n65 = property on="SyncStopEKG" class="Bool (strict)"("Val(Sgnl)"=FALSE ("Value (Signaling)")) -> ()  [unwired: 2 in, 2 out]
                n66 = property on="StartMeasureEKG" class="Bool"("DisabledEnum"=w154) -> ()  [unwired: 2 in, 2 out]
                n67 = property on="DeleteSignalEKG" class="Bool"("DisabledEnum"=w154) -> ()  [unwired: 2 in, 2 out]
                n68 = property on="SavePNG" class="Bool"("DisabledEnum"=w154) -> ()  [unwired: 2 in, 2 out]
                n69 = property on="Zobrazit graf č." class="DigNum (strict)"("DisabledEnum"=w154) -> ()  [unwired: 2 in, 2 out]
                n70 = property on="HintEKG" class="Bool"("DisabledEnum"=w154) -> ()  [unwired: 2 in, 2 out]
                n71 = property on="SaveCSV" class="Bool"("DisabledEnum"=w154) -> ()  [unwired: 2 in, 2 out]
                n72 = property on="UvodniStranka" class="Bool"("DisabledEnum"=w154) -> ()  [unwired: 2 in, 2 out]
                n73 = property on="ExitApp" class="Bool"("DisabledEnum"=w154) -> ()  [unwired: 2 in, 2 out]
                n74 = property on="UvodniStranka" class="Bool"("DisabledEnum"=T11."Enabled" ("Disabled")) -> ()  [unwired: 2 in, 2 out]
              }
              frame "ChangeTimeECG" {
                n75 = property on="EKGHRV" class="XYGraph (strict)"() -> ("XScale.Minimum"=w164:dbl)  [unwired: 2 in, 2 out]
                n76 = property on="GraphEKG" class="WFGraph (strict)"() -> ("XScale.Minimum"=w167:dbl)  [unwired: 2 in, 2 out]
                n77 = Add(x=w167, y="Délka časového okna (s)") -> (x+y=w166:dbl)
                n78 = Add(x=w164, y="Délka časového okna (s)") -> (x+y=w163:dbl)
                n79 = property on="GraphEKG" class="WFGraph (strict)"("XScale.Minimum"=w167, "XScale.Maximum"=w166) -> ()  [unwired: 2 in, 2 out]
                n80 = property on="EKGHRV" class="XYGraph (strict)"("XScale.Minimum"=w164, "XScale.Maximum"=w163) -> ()  [unwired: 2 in, 2 out]
              }
              frame "Exit" {
                n81 = flat-sequence {
                  frame #0 {
                  }
                  frame #1 {
                    n82 = property on="Tab Control" class="TabCtl (strict)"("Value"=T2."Uvod" ("Tab Control")) -> ()  [unwired: 2 in, 2 out]
                  }
                  frame #2 {
                    n83 = Stop(stop? (T)=TRUE) -> ()
                  }
                }
              }
              frame "Measure" {
                w176 = T11."Disabled and Grayed Out" ("Disabled")
                w192 = T14 16 items=["Flush Receive Buffer"=16, "Write Transmit Buffer to Device"=32, "Flush Receive Buffer (No I/O)"=64, "Flush Transmit Buffer"=128] ("Mask")
                w199 = T14 16 items=["Flush Receive Buffer"=16, "Write Transmit Buffer to Device"=32, "Flush Receive Buffer (No I/O)"=64, "Flush Transmit Buffer"=128] ("Mask")
                w217 = enum16{"1", "10", "100", "1000"}."1000" ("Sample Rate")
                n84 = case shown="\"1000\"" w217 {
                  tunnel: [1.0 10.0 100.0 1000.0] -> w190
                  frame "1", Default {
                  }
                  frame "10" {
                  }
                  frame "100" {
                  }
                  frame "1000" {
                  }
                }
                "Vzorkovacka" <- w190
                n85 = call-poly "VISA Configure Serial Port"("VISA resource name"="Vstupní COM port 2", "timeout (10sec)"=u32 2000, "baud rate (9600)"=u32 115200) -> ("VISA resource name out"=w226:refnum<visa-resource-name>, "error out"=w225:errorcluster)  [unwired: 11 in]
                n86 = Reciprocal(x=w190) -> (1/x=w207:dbl)
                n87 = property on="ChartEKG" class="WFChart (strict)"("XScale.Multiplier"=w207) -> ()  [unwired: 2 in, 2 out]
                n88 = call "InitBITalino.vi"("Battery \nThreshold (%)"=u8 5 ("Battery \nThreshold (%)"), "MODE"=FALSE, "error in (no error)"=w225, "Sample Rate"=w217, "BITalino"=w226) -> ("error out"=w194:errorcluster, "VISA out"=w196:refnum<visa-resource-name>)  [unwired: 4 in, 1 out]
                n89 = property on="StartMeasureEKG" class="Bool"("DisabledEnum"=w176) -> ()  [unwired: 2 in, 2 out]
                n90 = property on="DeleteSignalEKG" class="Bool"("DisabledEnum"=w176) -> ()  [unwired: 2 in, 2 out]
                n91 = property on="HintEKG" class="Bool"("DisabledEnum"=w176) -> ()  [unwired: 2 in, 2 out]
                n92 = property on="SaveCSV" class="Bool"("DisabledEnum"=w176) -> ()  [unwired: 2 in, 2 out]
                n93 = property on="SavePNG" class="Bool"("DisabledEnum"=w176) -> ()  [unwired: 2 in, 2 out]
                n94 = VISA Flush I/O Buffer(VISA resource name=w196, mask (16)=w192, error in (no error)=w194) -> (VISA resource name out=w195:refnum<visa-resource-name>, error out=w193:errorcluster)
                n95 = VISA Write(VISA resource name=w195, write buffer="0x03", error in (no error)=w193) -> (VISA resource name out=w211:refnum<visa-resource-name>, error out=w210:errorcluster)  [unwired: 1 out]
                n96 = while {
                  shift-right: [w252] -> w222
                  shift-left: w211 -> [w243]
                  shift-right: [w240] -> w212
                  shift-left: w210 -> [w242]
                  tunnel: [w246] -> w186 mode=indexing
                  shift-right: [FALSE] -> _
                  shift-left: TRUE -> [w239]
                  stop <- w237 stop-if-true
                  n97 = Equal?(x="Doba měření (s)", y=0.0) -> (x = y?=w236:bool)
                  n98 = case shown="True" w236 {
                    tunnel: w239 -> [_ w258]
                    tunnel: "Doba měření (s)" -> [_ w257]
                    tunnel: [w253 w255] -> w237
                    frame True {
                      n99 = local read "SyncStopEKG"() -> (w253:bool)
                    }
                    frame False {
                      n100 = call "Elapsed Time2"("Time Target (s)"=w257, "Reset"=w258) -> ("Time has Elapsed"=w256:bool)  [unwired: 10 in, 7 out]
                      n101 = local read "SyncStopEKG"() -> (w254:bool)
                      n102 = Or(x=w254, y=w256) -> (x .or. y?=w255:bool)
                    }
                  }
                  n103 = VISA Read(VISA resource name=w243, byte count=u32 8, error in (no error)=w242) -> (VISA resource name out=w252:refnum<visa-resource-name>, read buffer=w241:string, error out=w240:errorcluster)  [unwired: 1 out]
                  n104 = call "Packet Read.vi"("Packets"=w241) -> ("Analog Channels"=w247:cluster{u16, u16, u16, u16, u16, u16})  [unwired: 7 in, 3 out]
                  n105 = call "Conversion.vi"("Sensor Type"=T13 {"Sensor 1"=enum."ECG", "Sensor 2"=enum."ECG", "Sensor 3"=enum."ECG", "Sensor 4"=enum."ECG", "Sensor 5"=enum."ECG", "Sensor 6"=enum."ECG"}, "Analog Channels"=w247) -> ("output cluster"=w248:T15)  [unwired: 8 in, 1 out]
                  n106 = Cluster To Array(cluster=w248) -> (array=w251:dbl[])
                  n107 = Unbundle(w248) -> ("Result"=w246:dbl)  [unwired: 5 out]
                  n108 = Index Array(array=w251, index=2) -> (element=→"ChartEKG":dbl)
                }
                n109 = property on="Zobrazit graf č." class="DigNum (strict)"("DisabledEnum"=w176) -> ()  [unwired: 2 in, 2 out]
                n110 = property on="UvodniStranka" class="Bool"("DisabledEnum"=w176) -> ()  [unwired: 2 in, 2 out]
                n111 = property on="ExitApp" class="Bool"("DisabledEnum"=w176) -> ()  [unwired: 2 in, 2 out]
                n112 = Array Size(array=w186) -> (size(s)=w208:i32)
                n113 = Multiply(x=w208, y=w207) -> (x*y=w205:dbl)
                n114 = Reciprocal(x=w190) -> (1/x=w197:dbl)
                n115 = Round To Nearest(number=w205) -> (nearest integer value=w206:dbl)
                n116 = Build Array(u8 0) -> (w220:u8[])
                n117 = Build Array (concatenate)(w186, w185) -> (w183:dbl[][])
                n118 = Index Array(array=w183, index (row)=0) -> (element=w198:dbl[])  [unwired: 1 in]
                n119 = Bundle By Name("Y"=w198, "dt"=w197) -> (w216:waveform(dbl))  [unwired: 1 in]
                n120 = Build Array (concatenate)(w216, w187) -> (w188:waveform(dbl)[])
                n121 = Byte Array To String(unsigned byte array=w220) -> (string=w219:string)
                n122 = VISA Write(VISA resource name=w222, write buffer=w219, error in (no error)=w212) -> (VISA resource name out=w203:refnum<visa-resource-name>, error out=w201:errorcluster)  [unwired: 1 out]
                n123 = property on="GraphEKG" class="WFGraph (strict)"("XScale.Maximum"=w206) -> ()  [unwired: 2 in, 2 out]
                n124 = Index Array(array=w183, index (col)=0 ("index (row)")) -> (element=w182:dbl[])  [unwired: 1 in]
                n125 = VISA Flush I/O Buffer(VISA resource name=w203, mask (16)=w199, error in (no error)=w201) -> (VISA resource name out=w202:refnum<visa-resource-name>, error out=w200:errorcluster)
                n126 = Array Size(array=w182) -> (size(s)=w180:i32)
                "size(s) 3" <- w180
                n127 = Index Array(array=w188, index=0) -> (element=w189:waveform(dbl))
                "RawEKG" <- w189
                n128 = VISA Close(VISA resource name=w202, error in (no error)=w200) -> (error out=w204:errorcluster)
                n129 = call "RpeakDetector(subVI).vi"("Vstupní signál"=w189) -> ("Signál s peaky"=→"GraphEKG":waveform(dbl)[], "BPM"=→"BPM":i32, "XY-HRV"=→"EKGHRV":cluster{dbl[], dbl[]})
                n130 = Generate User Event(user event=w218, event data cluster=w204) -> ()  [unwired: 2 in, 2 out]
                n131 = property on="Zobrazit graf č." class="DigNum (strict)"("Maximum"=w180) -> ()  [unwired: 2 in, 2 out]
              }
              frame "Cursor" {
                n132 = local read "CoordsHRV"() -> (w266:T1)
                n133 = local read "CoordsEKG"() -> (w273:T1)
                n134 = invoke on="GraphEKG" class="WFGraph (strict)" method="Map Coords To XY"("Coords"=w273) -> ("XY"=w270:cluster{"X":dbl, "Y":dbl})  [unwired: 6 in, 6 out]
                n135 = invoke on="EKGHRV" class="XYGraph (strict)" method="Map Coords To XY"("Coords"=w266) -> ("XY"=w263:cluster{"X":dbl, "Y":dbl})  [unwired: 6 in, 6 out]
                n136 = Build Array (concatenate)(w270, w269) -> (w259:cluster{"X":dbl, "Y":dbl}[])
                n137 = Build Array (concatenate)(w263, w262) -> (w260:cluster{"X":dbl, "Y":dbl}[])
                n138 = property on="GraphEKG" class="WFGraph (strict)"("Cursor.Cursor Position"=w270, "Active Cursor"=u32 0, "Cursor.Allow Drag"=FALSE) -> ()  [unwired: 2 in, 2 out]
                n139 = property on="EKGHRV" class="XYGraph (strict)"("Cursor.Cursor Position"=w263, "Active Cursor"=u32 0, "Cursor.Allow Drag"=FALSE) -> ()  [unwired: 2 in, 2 out]
                n140 = property on="EKGxHRV" class="Bool (strict)"() -> ("Value"=w261:bool)  [unwired: 2 in, 2 out]
                n141 = case shown="True" w261 {
                  tunnel: w260 -> [_ w275]
                  tunnel: w259 -> [w274 _]
                  frame False {
                    n142 = local write "InfoCursor"(w274) -> ()
                  }
                  frame True {
                    "InfoCursor" <- w275
                  }
                }
              }
              frame "SaveCSV" {
                n143 = local read "RawEKG"() -> (w281:waveform(dbl))
                n144 = call "SaveFileToCSV(subVI).vi"("Typ signálu"="EKG (mV)", "Signál"=w281) -> ("error out"=→"error out 3":errorcluster)
              }
              frame "SavePNG" {
                n145 = control-ref of="GraphEKG"() -> (w288:refnum<vi>)
                n146 = call "SaveFileToBMP(subVI).vi"("WFGraph Refnum"=w288) -> ("error out"=→"error out 2":errorcluster)
              }
              frame "ShowGraphECG" {
                n147 = local read "Zobrazit graf č."() -> (w302:dbl)
                n148 = Index Array(array=w293, index (row)=w302) -> (element=w301:dbl[])  [unwired: 1 in]
                n149 = property on="Vzorkovacka" class="DigNum (strict)"() -> ("Value"=w295:dbl)  [unwired: 2 in, 2 out]
                n150 = Reciprocal(x=w295) -> (1/x=w294:dbl)
                n151 = Bundle By Name("Y"=w301, "dt"=w294) -> (w300:waveform(dbl))  [unwired: 1 in]
                n152 = Build Array(w300) -> (w296:waveform(dbl)[])
                n153 = Index Array(array=w296, index=0) -> (element=w299:waveform(dbl))
                n154 = call "RpeakDetector(subVI).vi"("Vstupní signál"=w299) -> ("Signál s peaky"=w298:waveform(dbl)[], "BPM"=w297:i32)  [unwired: 1 out]
                n155 = local write "GraphEKG"(w298) -> ()
                n156 = property on="BPM" class="DigNum (strict)"("Value"=w297) -> ()  [unwired: 2 in, 2 out]
              }
              frame "DeleteSignalEKG" {
                w308 = waveform(dbl) {"t0"=timestamp(0 s since 1904-01-01), "dt"=1.0, "Y"=[]} ("Waveform")
                n157 = property on="ChartEKG" class="WFChart (strict)"("History Data"=dbl[] []) -> ()  [unwired: 2 in, 2 out]
                n158 = local write "EKGHRV"(cluster{dbl[], dbl[]} {[], []} ("EKGHRV")) -> ()
                n159 = Build Array(w308, w308) -> (w307:waveform(dbl)[])
                n160 = local write "GraphEKG"(w307) -> ()
              }
              frame "HintEKG" {
                n161 = call "NapovedaEKG(subVI).vi"() -> ()  [unwired: 1 in]
              }
              frame "Intro" {
                n162 = property on="Tab Control" class="TabCtl (strict)"("Value"=T2."Uvod" ("Tab Control")) -> ()  [unwired: 2 in, 2 out]
              }
            }
          }
          frame Error {
          }
        }
      }
      frame "UlohaEEG" {
        n163 = case shown="Error .." w334 {
          tunnel: w339 -> [w351 _]
          tunnel: [w350 w519] -> w337
          tunnel: w336 -> [w349 w519]
          tunnel: w335 -> [w348 _]
          tunnel: [FALSE TRUE] -> w333
          tunnel: w330 -> [w346 w518]
          tunnel: [w345 w518] -> w329
          tunnel: w327 -> [w344 w517]
          tunnel: [w343 w517] -> w326
          tunnel: w325 -> [w342 w516]
          tunnel: [w341 w516] -> w324
          frame No Error {
            n164 = case shown="\"Measure\"" w351 {
              tunnel: [w356 w361 w376 w442 w461 w467 w474 w500 w504 w508 w514] -> w350
              tunnel: w349 -> [w356 w361 _ w442 w461 w467 w474 w500 w504 w508 w514]
              tunnel: w348 -> [_ _ w393 _ _ _ _ _ _ _ _]
              tunnel: w346 -> [w355 w360 w385 w443 w462 w468 w475 w499 w503 w507 w513]
              tunnel: [w355 w360 w374 w443 w462 w468 w475 w499 w503 w507 w513] -> w345
              tunnel: w344 -> [w353 w359 w366 w452 w460 w466 w473 w486 w502 w506 w512]
              tunnel: [w353 w359 w366 w445 w460 w466 w473 w486 w502 w506 w512] -> w343
              tunnel: w342 -> [w352 w358 w365 w447 w459 w465 w472 w485 w501 w505 w511]
              tunnel: [w352 w358 w365 w444 w459 w465 w472 w485 w501 w505 w511] -> w341
              frame "Wait", Default {
                n165 = property on="UvodniStranka" class="Bool"("DisabledEnum"=T11."Enabled" ("Disabled")) -> ()  [unwired: 2 in, 2 out]
                n166 = property on="SyncStopEEG" class="Bool (strict)"("Val(Sgnl)"=FALSE ("Value (Signaling)")) -> ()  [unwired: 2 in, 2 out]
              }
              frame "Exit" {
                n167 = flat-sequence {
                  frame #0 {
                    n168 = property on="Tab Control" class="TabCtl (strict)"("Value"=T2."Uvod" ("Tab Control")) -> ()  [unwired: 2 in, 2 out]
                    n169 = property on="ChartEEG" class="WFChart (strict)"("Visible"=TRUE) -> ()  [unwired: 2 in, 2 out]
                  }
                  frame #1 {
                    n170 = Stop(stop? (T)=TRUE) -> ()
                  }
                }
              }
              frame "Measure" {
                w388 = T14 16 items=["Flush Receive Buffer"=16, "Write Transmit Buffer to Device"=32, "Flush Receive Buffer (No I/O)"=64, "Flush Transmit Buffer"=128] ("Mask")
                w403 = enum16{"1", "10", "100", "1000"}."1000" ("Sample Rate")
                n171 = call-poly "VISA Configure Serial Port"("VISA resource name"="Vstupní COM port 4", "timeout (10sec)"=u32 2000, "baud rate (9600)"=u32 115200) -> ("VISA resource name out"=w411:refnum<visa-resource-name>, "error out"=w410:errorcluster)  [unwired: 11 in]
                n172 = case shown="\"1000\"" w403 {
                  tunnel: [1.0 10.0 100.0 1000.0] -> w377
                  frame "1", Default {
                  }
                  frame "10" {
                  }
                  frame "100" {
                  }
                  frame "1000" {
                  }
                }
                "vzorkovackaEEG" <- w377
                n173 = Reciprocal(x=w377) -> (1/x=w387:dbl)
                n174 = call "InitBITalino.vi"("Battery \nThreshold (%)"=u8 5 ("Battery \nThreshold (%)"), "MODE"=FALSE, "error in (no error)"=w410, "Sample Rate"=w403, "BITalino"=w411) -> ("error out"=w394:errorcluster, "VISA out"=w395:refnum<visa-resource-name>)  [unwired: 4 in, 1 out]
                n175 = VISA Write(VISA resource name=w395, write buffer="0x03", error in (no error)=w394) -> (VISA resource name out=w400:refnum<visa-resource-name>, error out=w399:errorcluster)  [unwired: 1 out]
                n176 = while {
                  shift-right: [w435] -> w407
                  shift-left: w400 -> [w425]
                  shift-right: [w427] -> w402
                  shift-left: w399 -> [w424]
                  tunnel: [w429] -> w384 mode=indexing
                  shift-right: [FALSE] -> _
                  shift-left: TRUE -> [w421]
                  stop <- w423 stop-if-true
                  n177 = case shown="0" "Doba měření (s)" {
                    tunnel: [w436 w439] -> w423
                    tunnel: "Doba měření (s)" -> [_ w441]
                    tunnel: w421 -> [_ w440]
                    frame 0 {
                      n178 = local read "SyncStopEEG"() -> (w436:bool)
                    }
                    frame Default {
                      n179 = call "Elapsed Time4"("Time Target (s)"=w441, "Reset"=w440) -> ("Time has Elapsed"=w438:bool)  [unwired: 10 in, 7 out]
                      n180 = local read "SyncStopEEG"() -> (w437:bool)
                      n181 = Or(x=w437, y=w438) -> (x .or. y?=w439:bool)
                    }
                  }
                  n182 = VISA Read(VISA resource name=w425, byte count=u32 8, error in (no error)=w424) -> (VISA resource name out=w435:refnum<visa-resource-name>, read buffer=w428:string, error out=w427:errorcluster)  [unwired: 1 out]
                  n183 = call "Packet Read.vi"("Packets"=w428) -> ("Analog Channels"=w430:cluster{u16, u16, u16, u16, u16, u16})  [unwired: 7 in, 3 out]
                  n184 = call "Conversion.vi"("Sensor Type"=T13 {"Sensor 1"=enum."EEG", "Sensor 2"=enum."EEG", "Sensor 3"=enum."EEG", "Sensor 4"=enum."EEG", "Sensor 5"=enum."EEG", "Sensor 6"=enum."EEG"}, "Analog Channels"=w430) -> ("output cluster"=w431:T15)  [unwired: 8 in, 1 out]
                  n185 = Cluster To Array(cluster=w431) -> (array=w434:dbl[])
                  n186 = Unbundle(w431) -> ("Result"=w429:dbl)  [unwired: 5 out]
                  n187 = Index Array(array=w434, index=2) -> (element=→"ChartEEG":dbl)
                }
                n188 = Reciprocal(x=w377) -> (1/x=w386:dbl)
                n189 = Build Array (concatenate)(w385, w384) -> (w374:dbl[][])
                n190 = Index Array(array=w374, index (row)="Zobrazit signál č._EEG") -> (element=w382:dbl[])  [unwired: 1 in]
                n191 = Bundle By Name("Y"=w382, "dt"=w386) -> (w381:waveform(dbl))  [unwired: 1 in]
                n192 = Build Array(w381) -> (w376:waveform(dbl)[])
                n193 = Index Array(array=w376, index=0) -> (element=w367:waveform(dbl))
                "RawEEG" <- w367
                n194 = Array Size(array=w384) -> (size(s)=w397:i32)
                n195 = Build Array(u8 0) -> (w405:u8[])
                n196 = call "EEGstats(subvi).vi"("Vstupní EEG"=w367) -> ("Beta vlny"=→"GraphEEG4":waveform(dbl), "Alpha vlny"=→"GraphEEG3":waveform(dbl), "Theta vlny"=→"GraphEEG2":waveform(dbl), "Delta vlny"=→"GraphEEG1":waveform(dbl))  [unwired: 1 in]
                n197 = Multiply(x=w397, y=w387) -> (x*y=w396:dbl)
                n198 = Byte Array To String(unsigned byte array=w405) -> (string=w404:string)
                n199 = VISA Write(VISA resource name=w407, write buffer=w404, error in (no error)=w402) -> (VISA resource name out=w390:refnum<visa-resource-name>, error out=w389:errorcluster)  [unwired: 1 out]
                n200 = VISA Flush I/O Buffer(VISA resource name=w390, mask (16)=w388, error in (no error)=w389) -> (VISA resource name out=w391:refnum<visa-resource-name>, error out=w392:errorcluster)
                n201 = Round To Nearest(number=w396) -> (nearest integer value=w380:dbl)
                n202 = Index Array(array=w374, index (col)=0 ("disabled index (col)")) -> (element=w372:dbl[])  [unwired: 1 in]
                n203 = VISA Close(VISA resource name=w391, error in (no error)=w392) -> (error out=w401:errorcluster)
                n204 = property on="GraphEEG2" class="WFGraph (strict)"("XScale.Maximum"=w380) -> ()  [unwired: 2 in, 2 out]
                n205 = property on="GraphEEG3" class="WFGraph (strict)"("XScale.Maximum"=w380) -> ()  [unwired: 2 in, 2 out]
                n206 = property on="GraphEEG4" class="WFGraph (strict)"("XScale.Maximum"=w380) -> ()  [unwired: 2 in, 2 out]
                n207 = property on="GraphEEG1" class="WFGraph (strict)"("XScale.Maximum"=w380) -> ()  [unwired: 2 in, 2 out]
                n208 = Array Size(array=w372) -> (size(s)=w375:i32)
                n209 = Generate User Event(user event=w393, event data cluster=w401) -> ()  [unwired: 2 in, 2 out]
                n210 = property on="Zobrazit signál č._EEG" class="DigNum (strict)"("Maximum"=w375) -> ()  [unwired: 2 in, 2 out]
              }
              frame "Cursor" {
                n211 = local read "CoordsEEGAlpha"() -> (w456:T1)
                n212 = local read "CoordsEEGBeta"() -> (w449:T1)
                n213 = invoke on="GraphEEG3" class="WFGraph (strict)" method="Map Coords To XY"("Coords"=w456) -> ("XY"=w453:cluster{"X":dbl, "Y":dbl})  [unwired: 6 in, 6 out]
                n214 = invoke on="GraphEEG4" class="WFGraph (strict)" method="Map Coords To XY"("Coords"=w449) -> ("XY"=w448:cluster{"X":dbl, "Y":dbl})  [unwired: 6 in, 6 out]
                n215 = Build Array (concatenate)(w453, w452) -> (w445:cluster{"X":dbl, "Y":dbl}[])
                n216 = Build Array (concatenate)(w448, w447) -> (w444:cluster{"X":dbl, "Y":dbl}[])
                n217 = property on="GraphEEG4" class="WFGraph (strict)"("Cursor.Cursor Position"=w448, "Active Cursor"=u32 0, "Cursor.Allow Drag"=FALSE) -> ()  [unwired: 2 in, 2 out]
                n218 = property on="GraphEEG3" class="WFGraph (strict)"("Cursor.Cursor Position"=w453, "Active Cursor"=u32 0, "Cursor.Allow Drag"=FALSE) -> ()  [unwired: 2 in, 2 out]
                n219 = property on="AlphaxBeta" class="Bool (strict)"() -> ("Value"=w446:bool)  [unwired: 2 in, 2 out]
                n220 = case shown="False" w446 {
                  tunnel: w445 -> [_ w458]
                  tunnel: w444 -> [w457 _]
                  frame False {
                    n221 = local write "InfoCursorEEG"(w457) -> ()
                  }
                  frame True {
                    "InfoCursorEEG" <- w458
                  }
                }
              }
              frame "SavePNG" {
                n222 = control-ref of="RawEEG"() -> (w464:refnum<vi>)
                n223 = call "SaveFileToBMP(subVI).vi"("WFGraph Refnum"=w464) -> ("error out"=→"error out 6":errorcluster)
              }
              frame "SaveCSV" {
                n224 = local read "RawEEG"() -> (w471:waveform(dbl))
                n225 = call "SaveFileToCSV(subVI).vi"("Typ signálu"="EEG (uV)", "Signál"=w471) -> ("error out"=→"error out 7":errorcluster)
              }
              frame "ChangeTimeEEG" {
                n226 = property on="GraphEEG2" class="WFGraph (strict)"() -> ("XScale.Minimum"=w482:dbl)  [unwired: 2 in, 2 out]
                n227 = property on="GraphEEG4" class="WFGraph (strict)"() -> ("XScale.Minimum"=w478:dbl)  [unwired: 2 in, 2 out]
                n228 = property on="GraphEEG1" class="WFGraph (strict)"() -> ("XScale.Minimum"=w484:dbl)  [unwired: 2 in, 2 out]
                n229 = property on="GraphEEG3" class="WFGraph (strict)"() -> ("XScale.Minimum"=w480:dbl)  [unwired: 2 in, 2 out]
                n230 = Add(x=w484, y="Časové okno všech signálů (s)") -> (x+y=w483:dbl)
                n231 = Add(x=w482, y="Časové okno všech signálů (s)") -> (x+y=w481:dbl)
                n232 = Add(x=w480, y="Časové okno všech signálů (s)") -> (x+y=w479:dbl)
                n233 = Add(x=w478, y="Časové okno všech signálů (s)") -> (x+y=w477:dbl)
                n234 = property on="GraphEEG1" class="WFGraph (strict)"("XScale.Minimum"=w484, "XScale.Maximum"=w483) -> ()  [unwired: 2 in, 2 out]
                n235 = property on="GraphEEG2" class="WFGraph (strict)"("XScale.Minimum"=w482, "XScale.Maximum"=w481) -> ()  [unwired: 2 in, 2 out]
                n236 = property on="GraphEEG3" class="WFGraph (strict)"("XScale.Minimum"=w480, "XScale.Maximum"=w479) -> ()  [unwired: 2 in, 2 out]
                n237 = property on="GraphEEG4" class="WFGraph (strict)"("XScale.Minimum"=w478, "XScale.Maximum"=w477) -> ()  [unwired: 2 in, 2 out]
              }
              frame "ShowGraphEEG" {
                n238 = local read "Zobrazit signál č._EEG"() -> (w498:dbl)
                n239 = Index Array(array=w499, index (row)=w498) -> (element=w497:dbl[])  [unwired: 1 in]
                n240 = property on="vzorkovackaEEG" class="DigNum (strict)"() -> ("Value"=w496:dbl)  [unwired: 2 in, 2 out]
                n241 = Reciprocal(x=w496) -> (1/x=w495:dbl)
                n242 = Bundle By Name("Y"=w497, "dt"=w495) -> (w494:waveform(dbl))  [unwired: 1 in]
                n243 = Build Array(w494) -> (w493:waveform(dbl)[])
                n244 = Index Array(array=w493, index=0) -> (element=w491:waveform(dbl))
                n245 = call "EEGstats(subvi).vi"("Vstupní EEG"=w491) -> ("Beta vlny"=w487:waveform(dbl), "Alpha vlny"=w488:waveform(dbl), "Theta vlny"=w489:waveform(dbl), "Delta vlny"=w490:waveform(dbl))  [unwired: 1 in]
                n246 = local write "GraphEEG1"(w490) -> ()
                n247 = local write "GraphEEG2"(w489) -> ()
                n248 = local write "GraphEEG3"(w488) -> ()
                n249 = local write "GraphEEG4"(w487) -> ()
              }
              frame "HintEEG" {
              }
              frame "DeleteSignal" {
                w509 = waveform(dbl) {"t0"=timestamp(0 s since 1904-01-01), "dt"=1.0, "Y"=[]} ("GraphEEG2")
                n250 = local write "GraphEEG2"(w509) -> ()
                n251 = local write "GraphEEG1"(w509) -> ()
                n252 = local write "GraphEEG4"(w509) -> ()
                n253 = local write "GraphEEG3"(w509) -> ()
                n254 = property on="ChartEEG" class="WFChart (strict)"("History Data"=dbl[] []) -> ()  [unwired: 2 in, 2 out]
              }
              frame "Intro" {
                n255 = property on="Tab Control" class="TabCtl (strict)"("Value"=T2."Uvod" ("Tab Control")) -> ()  [unwired: 2 in, 2 out]
              }
            }
          }
          frame Error {
          }
        }
      }
      frame "UlohaEDA" {
        n256 = case shown="\"Wait\", Default" w530 {
          frame "Wait", Default {
            n257 = property on="UvodniStranka" class="Bool"("DisabledEnum"=T11."Enabled" ("Disabled")) -> ()  [unwired: 2 in, 2 out]
          }
          frame "Exit" {
            n258 = flat-sequence {
              frame #0 {
                n259 = property on="Tab Control" class="TabCtl (strict)"("Value"=T2."Uvod" ("Tab Control")) -> ()  [unwired: 2 in, 2 out]
              }
              frame #1 {
                n260 = Stop(stop? (T)=TRUE) -> ()
              }
            }
          }
          frame "Measure" {
          }
          frame "Intro" {
            n261 = property on="Tab Control" class="TabCtl (strict)"("Value"=T2."Uvod" ("Tab Control")) -> ()  [unwired: 2 in, 2 out]
          }
          frame "UlohaEKG" {
          }
          frame "UlohaEMG" {
          }
          frame "PlaygroundMeas" {
          }
          frame "UlohaEEG" {
          }
          frame "UlohaEDA" {
          }
          frame "UlohaACC" {
          }
        }
      }
      frame "UlohaACC" {
        n262 = case shown="No Error" w543 {
          tunnel: w544 -> [w560 _]
          tunnel: w545 -> [w559 _]
          tunnel: [w558 w697] -> w539
          tunnel: w540 -> [w557 w697]
          tunnel: [FALSE TRUE] -> _
          tunnel: [w555 w695] -> w541
          tunnel: w542 -> [w554 w695]
          tunnel: w537 -> [w553 w694]
          tunnel: [w552 w694] -> w536
          frame No Error {
            n263 = case shown="\"Cursor\"" w560 {
              tunnel: w559 -> [_ _ _ _ w624 _ _ _ _ _ _]
              tunnel: [w565 w570 w574 w578 w599 w664 w671 w676 w685 w689 w693] -> w558
              tunnel: w557 -> [w565 w570 w574 w578 w588 w664 w671 w676 _ w689 w693]
              tunnel: [w563 w571 w573 w579 w595 w665 w672 w677 w684 w688 w692] -> w555
              tunnel: w554 -> [w563 w571 w573 w579 w597 w665 w672 w677 w684 w688 w692]
              tunnel: w553 -> [w562 w566 w572 w580 w585 w662 w668 w673 w682 w687 w690]
              tunnel: [w562 w566 w572 w577 w585 w662 w668 w673 w682 w687 w690] -> w552
              frame "Wait", Default {
                n264 = property on="UvodniStranka" class="Bool"("DisabledEnum"=T11."Enabled" ("Disabled")) -> ()  [unwired: 2 in, 2 out]
                n265 = property on="SyncStopACC" class="Bool (strict)"("Val(Sgnl)"=FALSE ("Value (Signaling)")) -> ()  [unwired: 2 in, 2 out]
              }
              frame "ChangeTimeACC" {
                n266 = property on="GraphACC" class="WFGraph (strict)"() -> ("XScale.Minimum"=w569:dbl)  [unwired: 2 in, 2 out]
                n267 = Add(x=w569, y="Délka časového okna (s) ACC") -> (x+y=w568:dbl)
                n268 = property on="GraphACC" class="WFGraph (strict)"("XScale.Minimum"=w569, "XScale.Maximum"=w568) -> ()  [unwired: 2 in, 2 out]
              }
              frame "Exit" {
                n269 = flat-sequence {
                  frame #0 {
                  }
                  frame #1 {
                    n270 = property on="Tab Control" class="TabCtl (strict)"("Value"=T2."Uvod" ("Tab Control")) -> ()  [unwired: 2 in, 2 out]
                  }
                  frame #2 {
                    n271 = Stop(stop? (T)=TRUE) -> ()
                  }
                }
              }
              frame "Cursor" {
                n272 = local read "CoordsACC"() -> (w584:T1)
                n273 = invoke on="GraphACC" class="WFGraph (strict)" method="Map Coords To XY"("Coords"=w584) -> ("XY"=w581:cluster{"X":dbl, "Y":dbl})  [unwired: 6 in, 6 out]
                n274 = Build Array (concatenate)(w581, w580) -> (w577:cluster{"X":dbl, "Y":dbl}[])
                "InfoCursorACC" <- w577
                n275 = property on="GraphACC" class="WFGraph (strict)"("Cursor.Cursor Position"=w581, "Active Cursor"=u32 0, "Cursor.Allow Drag"=FALSE) -> ()  [unwired: 2 in, 2 out]
              }
              frame "Measure" {
                w602 = T14 16 items=["Flush Receive Buffer"=16, "Write Transmit Buffer to Device"=32, "Flush Receive Buffer (No I/O)"=64, "Flush Transmit Buffer"=128] ("Mask")
                w609 = T14 16 items=["Flush Receive Buffer"=16, "Write Transmit Buffer to Device"=32, "Flush Receive Buffer (No I/O)"=64, "Flush Transmit Buffer"=128] ("Mask")
                w623 = enum16{"1", "10", "100", "1000"}."1000" ("Sample Rate")
                n276 = call-poly "VISA Configure Serial Port"("VISA resource name"="Vstupní COM port ACC", "timeout (10sec)"=u32 2000, "baud rate (9600)"=u32 115200) -> ("VISA resource name out"=w632:refnum<visa-resource-name>, "error out"=w631:errorcluster)  [unwired: 11 in]
                n277 = case shown="\"1000\"" w623 {
                  tunnel: [1.0 10.0 100.0 1000.0] -> w600
                  frame "1", Default {
                  }
                  frame "10" {
                  }
                  frame "100" {
                  }
                  frame "1000" {
                  }
                }
                "Vzorkovacka 2" <- w600
                n278 = Reciprocal(x=w600) -> (1/x=w592:dbl)
                n279 = property on="ChartACC" class="WFChart (strict)"("XScale.Multiplier"=w592) -> ()  [unwired: 2 in, 2 out]
                n280 = call "InitBITalino.vi"("Battery \nThreshold (%)"=u8 5 ("Battery \nThreshold (%)"), "MODE"=FALSE, "error in (no error)"=w631, "Sample Rate"=w623, "BITalino"=w632) -> ("error out"=w604:errorcluster, "VISA out"=w606:refnum<visa-resource-name>)  [unwired: 4 in, 1 out]
                n281 = VISA Flush I/O Buffer(VISA resource name=w606, mask (16)=w602, error in (no error)=w604) -> (VISA resource name out=w605:refnum<visa-resource-name>, error out=w603:errorcluster)
                n282 = VISA Write(VISA resource name=w605, write buffer="0x03", error in (no error)=w603) -> (VISA resource name out=w619:refnum<visa-resource-name>, error out=w618:errorcluster)  [unwired: 1 out]
                n283 = while {
                  shift-right: [w655] -> w628
                  shift-left: w619 -> [w647]
                  shift-right: [w644] -> w620
                  shift-left: w618 -> [w646]
                  tunnel: [w649] -> w598 mode=indexing
                  shift-right: [FALSE] -> _
                  shift-left: TRUE -> [w643]
                  stop <- w640 stop-if-true
                  n284 = case shown="0" "Doba měření (s) ACC" {
                    tunnel: w643 -> [_ w661]
                    tunnel: "Doba měření (s) ACC" -> [_ w660]
                    tunnel: [w656 w657] -> w640
                    frame 0 {
                      n285 = local read "SyncStopACC"() -> (w656:bool)
                    }
                    frame Default {
                      n286 = call "Elapsed Time5"("Time Target (s)"=w660, "Reset"=w661) -> ("Time has Elapsed"=w658:bool)  [unwired: 10 in, 7 out]
                      n287 = local read "SyncStopACC"() -> (w659:bool)
                      n288 = Or(x=w659, y=w658) -> (x .or. y?=w657:bool)
                    }
                  }
                  n289 = VISA Read(VISA resource name=w647, byte count=u32 8, error in (no error)=w646) -> (VISA resource name out=w655:refnum<visa-resource-name>, read buffer=w645:string, error out=w644:errorcluster)  [unwired: 1 out]
                  n290 = call "Packet Read.vi"("Packets"=w645) -> ("Analog Channels"=w650:cluster{u16, u16, u16, u16, u16, u16})  [unwired: 7 in, 3 out]
                  n291 = call "Conversion.vi"("Sensor Type"=T13 {"Sensor 1"=enum."ACC", "Sensor 2"=enum."ACC", "Sensor 3"=enum."ACC", "Sensor 4"=enum."ACC", "Sensor 5"=enum."ACC", "Sensor 6"=enum."ACC"}, "Analog Channels"=w650) -> ("output cluster"=w651:T15)  [unwired: 8 in, 1 out]
                  n292 = Cluster To Array(cluster=w651) -> (array=w654:dbl[])
                  n293 = Unbundle(w651) -> ("Result"=w649:dbl)  [unwired: 5 out]
                  n294 = Index Array(array=w654, index=2) -> (element=→"ChartACC":dbl)
                }
                n295 = Array Size(array=w598) -> (size(s)=w616:i32)
                n296 = Multiply(x=w616, y=w592) -> (x*y=w615:dbl)
                n297 = Reciprocal(x=w600) -> (1/x=w607:dbl)
                n298 = Round To Nearest(number=w615) -> (nearest integer value=w590:dbl)
                n299 = Build Array(u8 0) -> (w626:u8[])
                n300 = Build Array (concatenate)(w598, w597) -> (w595:dbl[][])
                n301 = Index Array(array=w595, index (row)=0) -> (element=w608:dbl[])  [unwired: 1 in]
                n302 = Bundle By Name("Y"=w608, "dt"=w607) -> (w622:waveform(dbl))  [unwired: 1 in]
                n303 = Build Array (concatenate)(w622, w588) -> (w599:waveform(dbl)[])
                n304 = Byte Array To String(unsigned byte array=w626) -> (string=w625:string)
                n305 = VISA Write(VISA resource name=w628, write buffer=w625, error in (no error)=w620) -> (VISA resource name out=w613:refnum<visa-resource-name>, error out=w611:errorcluster)  [unwired: 1 out]
                n306 = VISA Flush I/O Buffer(VISA resource name=w613, mask (16)=w609, error in (no error)=w611) -> (VISA resource name out=w612:refnum<visa-resource-name>, error out=w610:errorcluster)
                n307 = Index Array(array=w595, index (col)=0 ("index (row)")) -> (element=w594:dbl[])  [unwired: 1 in]
                n308 = property on="GraphACC" class="WFGraph (strict)"("XScale.Maximum"=w590) -> ()  [unwired: 2 in, 2 out]
                n309 = Array Size(array=w594) -> (size(s)=w589:i32)
                "size(s) 4" <- w589
                n310 = Index Array(array=w599, index=0) -> (element=w587:waveform(dbl))
                "RawACC" <- w587
                n311 = VISA Close(VISA resource name=w612, error in (no error)=w610) -> (error out=w614:errorcluster)
                n312 = Build Array(w587) -> (→"GraphACC":waveform(dbl)[])
                n313 = property on="Zobrazit signál č._ACC" class="DigNum (strict)"("Maximum"=w589) -> ()  [unwired: 2 in, 2 out]
                n314 = Generate User Event(user event=w624, event data cluster=w614) -> ()  [unwired: 2 in, 2 out]
              }
              frame "SaveCSV" {
                n315 = local read "RawACC"() -> (w666:waveform(dbl))
                n316 = call "SaveFileToCSV(subVI).vi"("Typ signálu"="ACC (g)", "Signál"=w666) -> ("error out"=→"error out 4":errorcluster)
              }
              frame "SavePNG" {
                n317 = control-ref of="GraphACC"() -> (w669:refnum<vi>)
                n318 = call "SaveFileToBMP(subVI).vi"("WFGraph Refnum"=w669) -> ("error out"=→"error out 5":errorcluster)
              }
              frame "ShowGraphACC" {
                n319 = Index Array(array=w677, index (row)="Zobrazit signál č._ACC") -> (element=w681:dbl[])  [unwired: 1 in]
                n320 = property on="Vzorkovacka 2" class="DigNum (strict)"() -> ("Value"=w679:dbl)  [unwired: 2 in, 2 out]
                n321 = Reciprocal(x=w679) -> (1/x=w678:dbl)
                n322 = Bundle By Name("Y"=w681, "dt"=w678) -> (w680:waveform(dbl))  [unwired: 1 in]
                n323 = Build Array(w680) -> (w674:waveform(dbl)[])
                n324 = local write "GraphACC"(w674) -> ()
              }
              frame "DeleteSignal" {
                w686 = waveform(dbl) {"t0"=timestamp(0 s since 1904-01-01), "dt"=1.0, "Y"=[]} ("Waveform")
                n325 = Build Array(w686, w686) -> (w685:waveform(dbl)[])
                n326 = property on="ChartACC" class="WFChart (strict)"("History Data"=dbl[] []) -> ()  [unwired: 2 in, 2 out]
                n327 = local write "GraphACC"(w685) -> ()
              }
              frame "HintACC" {
                n328 = call "NapovedaEKG(subVI).vi"() -> ()  [unwired: 1 in]
              }
              frame "Intro" {
                n329 = property on="Tab Control" class="TabCtl (strict)"("Value"=T2."Uvod" ("Tab Control")) -> ()  [unwired: 2 in, 2 out]
              }
            }
          }
          frame Error {
          }
        }
      }
      frame "UlohaEMG" {
        n330 = case shown="No Error" w707 {
          tunnel: w712 -> [w722 _]
          tunnel: w710 -> [w721 w865]
          tunnel: [w720 w865] -> w709
          tunnel: w708 -> [w719 _]
          tunnel: [FALSE TRUE] -> w706
          tunnel: w705 -> [w717 w864]
          tunnel: [w716 w864] -> w704
          tunnel: w699 -> [w715 w863]
          tunnel: [w714 w863] -> w698
          frame No Error {
            n331 = case shown="\"Measure\"" w722 {
              tunnel: w719 -> [_ _ _ w763 _ _ _ _ _ _ _ _]
              tunnel: w721 -> [w726 w730 w735 w742 w817 w832 w836 _ w846 w849 w856 w861]
              tunnel: [w726 w730 w735 w744 w817 w832 w836 w839 w846 w849 w856 w861] -> w720
              tunnel: w717 -> [w725 w729 w734 w745 w818 w831 w837 w840 w847 w850 w855 w860]
              tunnel: [w725 w729 w734 w739 w818 w831 w837 w840 w847 w850 w855 w860] -> w716
              tunnel: w715 -> [w724 w728 w733 w736 w820 w821 w833 w838 w842 w848 w854 w859]
              tunnel: [w724 w728 w733 w736 w819 w821 w833 w838 w842 w848 w854 w859] -> w714
              frame "Wait", Default {
                n332 = property on="UvodniStranka" class="Bool"("DisabledEnum"=T11."Enabled" ("Disabled")) -> ()  [unwired: 2 in, 2 out]
                n333 = property on="SyncStopEMG" class="Bool (strict)"("Val(Sgnl)"=FALSE ("SyncStopEMG")) -> ()  [unwired: 2 in, 2 out]
              }
              frame "Exit" {
                n334 = flat-sequence {
                  frame #0 {
                    n335 = property on="Tab Control" class="TabCtl (strict)"("Value"=T2."Uvod" ("Tab Control")) -> ()  [unwired: 2 in, 2 out]
                  }
                  frame #1 {
                    n336 = Stop(stop? (T)=TRUE) -> ()
                  }
                }
              }
              frame "HintEMG" {
                n337 = call "NapovedaEMG(subVI).vi"() -> ()  [unwired: 1 in]
              }
              frame "Measure" {
                w752 = T14 16 items=["Flush Receive Buffer"=16, "Write Transmit Buffer to Device"=32, "Flush Receive Buffer (No I/O)"=64, "Flush Transmit Buffer"=128] ("Mask")
                w757 = T14 16 items=["Flush Receive Buffer"=16, "Write Transmit Buffer to Device"=32, "Flush Receive Buffer (No I/O)"=64, "Flush Transmit Buffer"=128] ("Mask")
                w773 = enum16{"1", "10", "100", "1000"}."1000" ("Sample Rate")
                n338 = call-poly "VISA Configure Serial Port"("VISA resource name"="Vstupní COM port 3", "timeout (10sec)"=u32 2000, "baud rate (9600)"=u32 115200) -> ("VISA resource name out"=w782:refnum<visa-resource-name>, "error out"=w781:errorcluster)  [unwired: 11 in]
                n339 = case shown="\"1000\"" w773 {
                  tunnel: [1.0 10.0 100.0 1000.0] -> w774
                  frame "1", Default {
                  }
                  frame "10" {
                  }
                  frame "100" {
                  }
                  frame "1000" {
                  }
                }
                n340 = call "InitBITalino.vi"("Battery \nThreshold (%)"=u8 5 ("Battery \nThreshold (%)"), "MODE"=FALSE, "error in (no error)"=w781, "Sample Rate"=w773, "BITalino"=w782) -> ("error out"=w758:errorcluster, "VISA out"=w761:refnum<visa-resource-name>)  [unwired: 4 in, 1 out]
                n341 = Reciprocal(x=w774) -> (1/x=w750:dbl)
                n342 = VISA Flush I/O Buffer(VISA resource name=w761, mask (16)=w757, error in (no error)=w758) -> (VISA resource name out=w760:refnum<visa-resource-name>, error out=w759:errorcluster)
                n343 = property on="ChartEMG" class="WFChart (strict)"("XScale.Multiplier"=w750) -> ()  [unwired: 2 in, 2 out]
                n344 = VISA Write(VISA resource name=w760, write buffer="0x03", error in (no error)=w759) -> (VISA resource name out=w768:refnum<visa-resource-name>, error out=w767:errorcluster)  [unwired: 1 out]
                n345 = while {
                  shift-right: [w806] -> w778
                  shift-left: w768 -> [w796]
                  shift-right: [w798] -> w770
                  shift-left: w767 -> [w795]
                  tunnel: [w800] -> w748 mode=indexing
                  shift-right: [FALSE] -> _
                  shift-left: TRUE -> [w793]
                  stop <- w790 stop-if-true
                  n346 = case shown="0" "Doba měření (s)" {
                    tunnel: "Doba měření (s)" -> [_ w811]
                    tunnel: w793 -> [_ w812]
                    tunnel: [w807 w809] -> w790
                    frame 0 {
                      n347 = local read "SyncStopEMG"() -> (w807:bool)
                    }
                    frame Default {
                      n348 = call "Elapsed Time3"("Time Target (s)"=w811, "Reset"=w812) -> ("Time has Elapsed"=w810:bool)  [unwired: 10 in, 7 out]
                      n349 = local read "SyncStopEMG"() -> (w808:bool)
                      n350 = Or(x=w808, y=w810) -> (x .or. y?=w809:bool)
                    }
                  }
                  n351 = VISA Read(VISA resource name=w796, byte count=u32 8, error in (no error)=w795) -> (VISA resource name out=w806:refnum<visa-resource-name>, read buffer=w799:string, error out=w798:errorcluster)  [unwired: 1 out]
                  n352 = call "Packet Read.vi"("Packets"=w799) -> ("Analog Channels"=w801:cluster{u16, u16, u16, u16, u16, u16})  [unwired: 7 in, 3 out]
                  n353 = call "Conversion.vi"("Sensor Type"=T13 {"Sensor 1"=enum."EMG", "Sensor 2"=enum."EMG", "Sensor 3"=enum."EMG", "Sensor 4"=enum."EMG", "Sensor 5"=enum."EMG", "Sensor 6"=enum."EMG"}, "Analog Channels"=w801) -> ("output cluster"=w802:T15)  [unwired: 8 in, 1 out]
                  n354 = Cluster To Array(cluster=w802) -> (array=w805:dbl[])
                  n355 = Unbundle(w802) -> ("Result"=w800:dbl)  [unwired: 5 out]
                  n356 = Index Array(array=w805, index=2) -> (element=→"ChartEMG":dbl)
                }
                n357 = Reciprocal(x=w774) -> (1/x=w746:dbl)
                n358 = Array Size(array=w748) -> (size(s)=w765:i32)
                n359 = Build Array(u8 0) -> (w776:u8[])
                n360 = Multiply(x=w765, y=w750) -> (x*y=w764:dbl)
                n361 = Byte Array To String(unsigned byte array=w776) -> (string=w775:string)
                n362 = VISA Write(VISA resource name=w778, write buffer=w775, error in (no error)=w770) -> (VISA resource name out=w754:refnum<visa-resource-name>, error out=w753:errorcluster)  [unwired: 1 out]
                n363 = Round To Nearest(number=w764) -> (nearest integer value=w749:dbl)
                n364 = Build Array (concatenate)(w745, w748) -> (w739:dbl[][])
                n365 = Index Array(array=w739, index (row)="Zobrazit signál č.") -> (element=w747:dbl[])  [unwired: 1 in]
                n366 = Bundle By Name("Y"=w747, "dt"=w746) -> (w772:waveform(dbl))  [unwired: 1 in]
                n367 = Build Array (concatenate)(w772, w742) -> (w744:waveform(dbl)[])
                n368 = property on="GraphEMG" class="WFGraph (strict)"("XScale.Maximum"=w749) -> ()  [unwired: 2 in, 2 out]
                n369 = VISA Flush I/O Buffer(VISA resource name=w754, mask (16)=w752, error in (no error)=w753) -> (VISA resource name out=w755:refnum<visa-resource-name>, error out=w756:errorcluster)
                n370 = Index Array(array=w744, index=0) -> (element=w737:waveform(dbl))
                "RawEMG" <- w737
                n371 = VISA Close(VISA resource name=w755, error in (no error)=w756) -> (error out=w769:errorcluster)
                n372 = call "EMGstats(subvi).vi"("EMG signál"=w737) -> ("Signál s vlastnostmi"=→"GraphEMG":waveform(dbl)[])  [unwired: 1 in, 1 out]
                n373 = Index Array(array=w739, index (col)=0 ("index (row)")) -> (element=w741:dbl[])  [unwired: 1 in]
                n374 = Generate User Event(user event=w763, event data cluster=w769) -> ()  [unwired: 2 in, 2 out]
                n375 = Array Size(array=w741) -> (size(s)=w738:i32)
                n376 = property on="Zobrazit signál č." class="DigNum (strict)"("Maximum"=w738) -> ()  [unwired: 2 in, 2 out]
              }
              frame "Cursor" {
                n377 = local read "CoordsEMG"() -> (w816:T1)
                n378 = invoke on="GraphEMG" class="WFGraph (strict)" method="Map Coords To XY"("Coords"=w816) -> ("XY"=w815:cluster{"X":dbl, "Y":dbl})  [unwired: 6 in, 6 out]
                n379 = Build Array (concatenate)(w815, w820) -> (w819:cluster{"X":dbl, "Y":dbl}[])
                "InfoCursorEMG" <- w819
                n380 = property on="GraphEMG" class="WFGraph (strict)"("Cursor.Cursor Position"=w815, "Active Cursor"=u32 0, "Cursor.Allow Drag"=FALSE) -> ()  [unwired: 2 in, 2 out]
              }
              frame "ShowGraphEMG" {
                n381 = local read "Zobrazit signál č."() -> (w830:dbl)
                n382 = Index Array(array=w831, index (row)=w830) -> (element=w829:dbl[])  [unwired: 1 in]
                n383 = Reciprocal(x=1000.0) -> (1/x=w828:dbl)
                n384 = Bundle By Name("Y"=w829, "dt"=w828) -> (w826:waveform(dbl))  [unwired: 1 in]
                n385 = Build Array(w826) -> (w825:waveform(dbl)[])
                n386 = Index Array(array=w825, index=0) -> (element=w823:waveform(dbl))
                n387 = call "EMGstats(subvi).vi"("EMG signál"=w823) -> ("Signál s vlastnostmi"=w822:waveform(dbl)[])  [unwired: 1 in, 1 out]
                n388 = local write "GraphEMG"(w822) -> ()
              }
              frame "SavePNG" {
                n389 = control-ref of="GraphEMG"() -> (w835:refnum<vi>)
                n390 = call "SaveFileToBMP(subVI).vi"("WFGraph Refnum"=w835) -> ("error out"=→"error out":errorcluster)
              }
              frame "DeleteSignal" {
                w839 = waveform(dbl)[] [] ("GraphEMG")
                n391 = property on="ChartEMG" class="WFChart (strict)"("History Data"=dbl[] []) -> ()  [unwired: 2 in, 2 out]
                n392 = local write "GraphEMG"(w839) -> ()
              }
              frame "SaveCSV" {
                n393 = local read "RawEMG"() -> (w844:waveform(dbl))
                n394 = call "SaveFileToCSV(subVI).vi"("Typ signálu"="EMG (mV)", "Signál"=w844) -> ("error out"=w845:errorcluster)
                n395 = local write "error out 3"(w845) -> ()
              }
              frame "ChangeTimeEMG" {
                n396 = property on="GraphEMG" class="WFGraph (strict)"() -> ("XScale.Minimum"=w851:dbl)  [unwired: 2 in, 2 out]
                n397 = Add(x=w851, y="Délka časového okna (s) EMG") -> (x+y=w852:dbl)
                n398 = property on="GraphEMG" class="WFGraph (strict)"("XScale.Minimum"=w851, "XScale.Maximum"=w852) -> ()  [unwired: 2 in, 2 out]
              }
              frame "DeleteSignalEMG" {
                n399 = property on="ChartEMG" class="WFChart (strict)"("History Data"=dbl[] []) -> ()  [unwired: 2 in, 2 out]
                n400 = local write "GraphEMG"(waveform(dbl)[] [] ("GraphEMG")) -> ()
              }
              frame "Intro" {
                n401 = property on="Tab Control" class="TabCtl (strict)"("Value"=T2."Uvod" ("Tab Control")) -> ()  [unwired: 2 in, 2 out]
              }
            }
          }
          frame Error {
          }
        }
      }
      frame "PlaygroundMeas" {
        n402 = case shown="No Error" w878 {
          tunnel: w880 -> [w885 _]
          tunnel: [FALSE TRUE] -> w875
          tunnel: w879 -> [w883 _]
          tunnel: [w882 w981] -> w874
          tunnel: w871 -> [w881 w981]
          frame No Error {
            n403 = case shown="\"Measure\"" w885 {
              tunnel: w883 -> [_ _ _ _ w920 _]
              tunnel: [w886 w889 w895 w897 w900 w978] -> w882
              tunnel: w881 -> [w886 w889 w895 w897 _ w978]
              frame "Wait", Default {
                n404 = property on="UvodniStranka" class="Bool"("DisabledEnum"=T11."Enabled" ("Disabled")) -> ()  [unwired: 2 in, 2 out]
                n405 = property on="SyncStop" class="Bool (strict)"("Val(Sgnl)"=FALSE ("Value (Signaling)")) -> ()  [unwired: 2 in, 2 out]
              }
              frame "Exit" {
                n406 = flat-sequence {
                  frame #0 {
                    w891 = waveform(dbl) {"t0"=timestamp(0 s since 1904-01-01), "dt"=1.0, "Y"=[0.0]} ("Waveform")
                    n407 = property on="Tab Control" class="TabCtl (strict)"("Value"=T2."Uvod" ("Tab Control")) -> ()  [unwired: 2 in, 2 out]
                    n408 = Build Array(w891, w891) -> (w890:waveform(dbl)[])
                    n409 = call-poly <vilib>:"FFT Spectrum (Mag-Phase).vi"("time signals"=w890) -> ("magnitudes"=w892:cluster{"f0":dbl, "df":dbl, "magnitude":dbl[]}[])  [unwired: 6 in, 4 out]
                    n410 = local write "SpectrumPlayground"(w892) -> ()
                    n411 = property on="Waveform Graph" class="WFGraph (strict)"("Value"=w890) -> ()  [unwired: 2 in, 2 out]
                  }
                  frame #1 {
                    n412 = Stop(stop? (T)=TRUE) -> ()
                  }
                }
              }
              frame "PlaygroundFiltr" {
                n413 = property on="Tab Control" class="TabCtl (strict)"("Value"=T2."PlaygroundFiltr" ("Tab Control")) -> ()  [unwired: 2 in, 2 out]
              }
              frame "Intro" {
                n414 = flat-sequence {
                  frame #0 {
                    n415 = property on="Tab Control" class="TabCtl (strict)"("Value"=T2."Uvod" ("Tab Control")) -> ()  [unwired: 2 in, 2 out]
                  }
                  frame #1 {
                    n416 = Wait (ms)(milliseconds to wait=u32 100) -> ()  [unwired: 1 out]
                  }
                }
              }
              frame "Measure" {
                w905 = T14 16 items=["Flush Receive Buffer"=16, "Write Transmit Buffer to Device"=32, "Flush Receive Buffer (No I/O)"=64, "Flush Transmit Buffer"=128] ("Mask")
                w922 = "Signal" ("name (unnamed)")
                n417 = property on="Vzorkovací frekvence (Hz)" class="Enum (strict)"() -> ("Value"=w917:enum16{"1", "10", "100", "1000"})  [unwired: 2 in, 2 out]
                n418 = call-poly "VISA Configure Serial Port"("VISA resource name"="Vstupní COM port", "timeout (10sec)"=u32 2000, "baud rate (9600)"=u32 115200) -> ("VISA resource name out"=w933:refnum<visa-resource-name>, "error out"=w932:errorcluster)  [unwired: 11 in]
                n419 = case shown="\"1000\"" w917 {
                  tunnel: [1.0 10.0 100.0 1000.0] -> w915
                  frame "1", Default {
                  }
                  frame "10" {
                  }
                  frame "100" {
                  }
                  frame "1000" {
                  }
                }
                n420 = Reciprocal(x=w915) -> (1/x=w902:dbl)
                n421 = call "InitBITalino.vi"("Battery \nThreshold (%)"=u8 5 ("Battery \nThreshold (%)"), "MODE"=FALSE, "error in (no error)"=w932, "Sample Rate"="Vzorkovací frekvence (Hz)", "BITalino"=w933) -> ("error out"=w929:errorcluster, "VISA out"=w913:refnum<visa-resource-name>)  [unwired: 4 in, 1 out]
                n422 = property on="Waveform Chart" class="WFChart (strict)"("XScale.Multiplier"=w902) -> ()  [unwired: 2 in, 2 out]
                n423 = Obtain Queue(name (unnamed)=w922, element data type=w922, error in (no error)=w929) -> (queue out=w921:refnum<queue>, error out=w912:errorcluster)  [unwired: 2 in, 1 out]
                n424 = VISA Write(VISA resource name=w913, write buffer="0x03", error in (no error)=w912) -> (VISA resource name out=w910:refnum<visa-resource-name>, error out=w911:errorcluster)  [unwired: 1 out]
                n425 = while {
                  shift-right: [w975] -> w928
                  shift-left: w910 -> [w964]
                  shift-right: [w970] -> w916
                  shift-left: w911 -> [w965]
                  shift-right: [w971] -> w926
                  shift-left: w921 -> [w974]
                  stop <- w969 stop-if-true
                  n426 = call "Elapsed Time"("Time Target (s)"="Time Target (s)") -> ("Time has Elapsed"=w967:bool)  [unwired: 11 in, 7 out]
                  n427 = VISA Read(VISA resource name=w964, byte count=u32 8, error in (no error)=w965) -> (VISA resource name out=w975:refnum<visa-resource-name>, read buffer=w973:string, error out=w972:errorcluster)  [unwired: 1 out]
                  n428 = Enqueue Element(queue=w974, element=w973, error in (no error)=w972) -> (queue out=w971:refnum<queue>, error out=w970:errorcluster)  [unwired: 1 in, 1 out]
                  n429 = Unbundle By Name(w970) -> ("status"=w968:bool)
                  n430 = Or(x=w968, y=w967) -> (x .or. y?=w969:bool)
                }
                n431 = while {
                  tunnel: w921 -> [w953]
                  tunnel: "Cluster" -> [w949]
                  tunnel: [w947] -> w903
                  stop <- w950 stop-if-true
                  n432 = Dequeue Element(queue=w953) -> (element=w952:string, error out=w951:errorcluster)  [unwired: 2 in, 2 out]
                  n433 = case shown="No Error" w951 {
                    tunnel: w952 -> [w961 _]
                    tunnel: [FALSE TRUE] -> w950
                    tunnel: w949 -> [w956 _]
                    tunnel: [w954 w962] -> w948
                    frame No Error {
                      n434 = Cluster To Array(cluster=w956) -> ()  [unwired: 1 out]
                      n435 = call "Packet Read.vi"("Packets"=w961) -> ("Analog Channels"=w960:cluster{u16, u16, u16, u16, u16, u16})  [unwired: 7 in, 3 out]
                      n436 = call "Conversion.vi"("Sensor Type"="Druh signálu", "Analog Channels"=w960) -> ("output cluster"=w955:T15)  [unwired: 8 in, 1 out]
                      n437 = Cluster To Array(cluster=w955) -> (array=→"Waveform Chart":dbl[])
                      n438 = Cluster To Array(cluster=w955) -> (array=w954:dbl[])
                      "array" <- w954
                    }
                    frame Error {
                      n439 = local read "array"() -> (w962:dbl[])
                    }
                  }
                  n440 = Build Array(w948) -> (w947:dbl[][])
                }
                n441 = Build Array(u8 0) -> (w924:u8[])
                n442 = Byte Array To String(unsigned byte array=w924) -> (string=w923:string)
                n443 = VISA Write(VISA resource name=w928, write buffer=w923, error in (no error)=w916) -> (VISA resource name out=w909:refnum<visa-resource-name>, error out=w907:errorcluster)  [unwired: 1 out]
                n444 = VISA Flush I/O Buffer(VISA resource name=w909, mask (16)=w905, error in (no error)=w907) -> (VISA resource name out=w908:refnum<visa-resource-name>, error out=w906:errorcluster)
                n445 = for {
                  N: 5 -> [_]
                  tunnel: w903 -> [w942]
                  tunnel: w902 -> [w939]
                  tunnel: [w937] -> w900
                  i -> [w941]
                  n446 = Index Array(array=w942, index (row)=w941) -> (element=w940:dbl[])  [unwired: 1 in]
                  n447 = Bundle By Name("Y"=w940, "dt"=w939) -> (w938:waveform(dbl))  [unwired: 1 in]
                  n448 = Build Array(w938) -> (w937:waveform(dbl)[])
                }
                "Waveform" <- w900
                n449 = VISA Close(VISA resource name=w908, error in (no error)=w906) -> (error out=w927:errorcluster)
                n450 = Release Queue(queue=w926, error in (no error)=w927) -> (error out=w919:errorcluster)  [unwired: 1 in, 2 out]
                n451 = Generate User Event(user event=w920, event data cluster=w919) -> ()  [unwired: 2 in, 2 out]
              }
              frame "DeleteSignal" {
                n452 = property on="Waveform Chart" class="WFChart (strict)"("History Data"=dbl[] []) -> ()  [unwired: 2 in, 2 out]
                n453 = local write "Waveform"(waveform(dbl)[] [] ("Waveform")) -> ()
              }
            }
          }
          frame Error {
          }
        }
      }
    }
  }
  n454 = while {
    shift-right: [w987] -> w15
    shift-left: w19 -> [w986]
    shift-right: [w988] -> w16
    shift-left: w20 -> [w989]
    tunnel: [w984] -> w13
    tunnel: w9 -> [w983]
    stop <- w982 stop-if-true
    n455 = event shown="[32] \"GraphEEG3\": Mouse Down" {
      selector: w983 -> [_ _ _ _ _ _ _ _ _ _ _ _ _ _ _ _ _ _ _ _ _ _ _ _ _ _ _ _ _ _ _ _ _ _ _ _ _ _ _ _ _ _ _ _ _ _ _ _ _ _ _ _ _ _ _]
      dyn-events: [_ _ _ _ _ _ _ _ _ _ _ _ _ _ _ _ _ _ _ _ _ _ _ _ _ _ _ _ _ _ _ _ _ _ _ _ _ _ _ _ _ _ _ _ _ _ _ _ _ _ _ _ _ _ _] -> w984
      timeout: _ -> [_ _ _ _ _ _ _ _ _ _ _ _ _ _ _ _ _ _ _ _ _ _ _ _ _ _ _ _ _ _ _ _ _ _ _ _ _ _ _ _ _ _ _ _ _ _ _ _ _ _ _ _ _ _ _]
      tunnel: w989 -> [_ w995 w1000 w1008 w1016 w1024 w1032 w1043 w1051 w1059 w1064 w1075 w1086 w1097 w1113 w1117 w1122 w1131 w1139 w1147 w1155 w1169 _ w1178 w1186 w1194 w1202 w1210 w1218 w1226 w1235 w1244 w1254 w1264 w1273 w1283 w1292 w1300 w1308 w1316 w1324 w1332 w1343 w1351 w1362 w1370 w1375 w1386 w1394 w1399 w1407 w1415 w1423 w1431 w1439]
      tunnel: w986 -> [_ w994 w998 w1007 w1015 w1023 w1031 w1042 w1050 w1058 w1062 w1073 w1084 w1095 w1112 w1116 w1121 w1130 w1138 w1146 w1154 w1168 _ w1176 w1185 w1193 w1201 w1209 w1217 w1225 w1234 w1243 w1253 w1263 w1272 w1282 w1291 w1299 w1307 w1315 w1323 w1331 w1342 w1350 w1361 w1369 w1373 w1385 w1393 w1398 w1404 w1412 w1420 w1428 w1436]
      tunnel: [_ w993 w999 w1004 w1012 w1020 w1027 w1035 w1048 w1053 w1069 w1080 w1091 w1102 w1109 w1117 w1122 w1124 w1133 w1141 w1149 w1159 _ w1173 w1182 w1190 w1199 w1206 w1214 w1222 w1230 w1239 w1249 w1259 w1268 w1278 w1288 w1294 w1304 w1312 w1320 w1328 w1341 w1348 w1360 w1367 w1378 w1382 w1390 w1397 w1405 w1413 w1421 w1429 w1437] -> w988
      tunnel: [_ w992 w997 w1002 w1011 w1018 w1026 w1034 w1046 w1055 w1066 w1077 w1088 w1099 w1105 w1116 w1121 w1125 w1134 w1142 w1150 w1157 _ w1172 w1180 w1188 w1197 w1204 w1212 w1221 w1229 w1238 w1248 w1258 w1267 w1277 w1287 w1293 w1303 w1310 w1319 w1327 w1340 w1347 w1359 w1365 w1377 w1380 w1388 w1396 w1402 w1410 w1418 w1426 w1434] -> w987
      tunnel: [_ w990 _ _ _ _ _ _ _ _ _ _ _ _ _ _ _ _ _ _ _ _ _ _ _ _ _ _ _ _ _ _ _ _ _ _ _ _ _ _ _ _ _ _ _ _ _ _ _ _ _ _ _ _ _] -> w982
      event Timeout {
        n456 = event-data() -> ()  [unwired: 1 in, 3 out]
      }
      event "ExitApp": Value Change {
        w990 = TRUE
        n457 = event-data() -> ()  [unwired: 1 in, 6 out]
        n458 = Enqueue Element(queue=w995, element=enum16{"Wait", "Exit", "Measure"}."Exit", error in (no error)=w994) -> (queue out=w993:refnum<queue>, error out=w992:errorcluster)  [unwired: 1 in, 1 out]
        n459 = property on="Tab Control" class="TabCtl (strict)"("Tabs Visible?"=w990) -> ()  [unwired: 2 in, 2 out]
      }
      event "OdstranitFiltr": Value Change {
        n460 = event-data() -> ()  [unwired: 1 in, 6 out]
        n461 = Enqueue Element(queue=w1000, element=T16."RemoveFilter", error in (no error)=w998) -> (queue out=w999:refnum<queue>, error out=w997:errorcluster)  [unwired: 1 in, 1 out]
      }
      event "UlohaEEG": Value Change {
        n462 = event-data() -> ()  [unwired: 1 in, 6 out]
        n463 = Enqueue Element(queue=w1008, element=T17."UlohaEEG", error in (no error)=w1007) -> (queue out=w1005:refnum<queue>, error out=w1003:errorcluster)  [unwired: 1 in, 1 out]
        n464 = Enqueue Element(queue=w1005, element=T17."Wait", error in (no error)=w1003) -> (queue out=w1004:refnum<queue>, error out=w1002:errorcluster)  [unwired: 1 in, 1 out]
      }
      event "UlohaEMG": Value Change {
        n465 = event-data() -> ()  [unwired: 1 in, 6 out]
        n466 = Enqueue Element(queue=w1016, element=T18."UlohaEMG", error in (no error)=w1015) -> (queue out=w1013:refnum<queue>, error out=w1010:errorcluster)  [unwired: 1 in, 1 out]
        n467 = Enqueue Element(queue=w1013, element=T18."Wait", error in (no error)=w1010) -> (queue out=w1012:refnum<queue>, error out=w1011:errorcluster)  [unwired: 1 in, 1 out]
      }
      event "UlohaEKG": Value Change {
        n468 = event-data() -> ()  [unwired: 1 in, 6 out]
        n469 = Enqueue Element(queue=w1024, element=T19."UlohaEKG", error in (no error)=w1023) -> (queue out=w1021:refnum<queue>, error out=w1019:errorcluster)  [unwired: 1 in, 1 out]
        n470 = Enqueue Element(queue=w1021, element=T19."Wait", error in (no error)=w1019) -> (queue out=w1020:refnum<queue>, error out=w1018:errorcluster)  [unwired: 1 in, 1 out]
      }
      event "UvodniStranka": Value Change {
        n471 = event-data() -> ()  [unwired: 1 in, 6 out]
        n472 = Enqueue Element(queue=w1032, element=T19."Intro", error in (no error)=w1031) -> (queue out=w1029:refnum<queue>, error out=w1028:errorcluster)  [unwired: 1 in, 1 out]
        n473 = Enqueue Element(queue=w1029, element=T19."Wait", error in (no error)=w1028) -> (queue out=w1027:refnum<queue>, error out=w1026:errorcluster)  [unwired: 1 in, 1 out]
      }
      event "StartMeasureACC": Value Change {
        n474 = event-data() -> ()  [unwired: 1 in, 6 out]
        n475 = Enqueue Element(queue=w1043, element=T20."UlohaACC", error in (no error)=w1042) -> (queue out=w1040:refnum<queue>, error out=w1039:errorcluster)  [unwired: 1 in, 1 out]
        n476 = Enqueue Element(queue=w1040, element=T20."DeleteSignal", error in (no error)=w1039) -> (queue out=w1037:refnum<queue>, error out=w1036:errorcluster)  [unwired: 1 in, 1 out]
        n477 = Enqueue Element(queue=w1037, element=T20."Measure", error in (no error)=w1036) -> (queue out=w1035:refnum<queue>, error out=w1034:errorcluster)  [unwired: 1 in, 1 out]
      }
      event "UlohaACC": Value Change {
        n478 = event-data() -> ()  [unwired: 1 in, 6 out]
        n479 = Enqueue Element(queue=w1051, element=T17."UlohaACC", error in (no error)=w1050) -> (queue out=w1049:refnum<queue>, error out=w1047:errorcluster)  [unwired: 1 in, 1 out]
        n480 = Enqueue Element(queue=w1049, element=T17."Wait", error in (no error)=w1047) -> (queue out=w1048:refnum<queue>, error out=w1046:errorcluster)  [unwired: 1 in, 1 out]
      }
      event "Playground": Value Change {
        n481 = event-data() -> ()  [unwired: 1 in, 6 out]
        n482 = Enqueue Element(queue=w1059, element=T18."PlaygroundMeas", error in (no error)=w1058) -> (queue out=w1054:refnum<queue>, error out=w1056:errorcluster)  [unwired: 1 in, 1 out]
        n483 = Enqueue Element(queue=w1054, element=T18."Wait", error in (no error)=w1056) -> (queue out=w1053:refnum<queue>, error out=w1055:errorcluster)  [unwired: 1 in, 1 out]
      }
      event "StopMeasure": Value Change {
        n484 = event-data() -> ()  [unwired: 1 in, 6 out]
        n485 = Enqueue Element(queue=w1064, element=T18."PlaygroundMeas", error in (no error)=w1062) -> (queue out=w1063:refnum<queue>, error out=w1061:errorcluster)  [unwired: 1 in, 1 out]
        n486 = property on="SyncStop" class="Bool (strict)"("Visible"=FALSE) -> ()  [unwired: 2 in, 2 out]
        n487 = Enqueue Element(queue=w1063, element=enum16{"Wait", "Exit", "Measure"}."Wait", error in (no error)=w1061) -> (queue out=w1069:refnum<queue>, error out=w1067:errorcluster)  [unwired: 1 in, 1 out]
        n488 = property on="SyncStop" class="Bool (strict)"(error in=w1067, "Val(Sgnl)"=TRUE ("Value (Signaling)")) -> (error out=w1066:errorcluster)  [unwired: 1 in, 1 out]
      }
      event "StopMeasureEMG": Value Change {
        n489 = event-data() -> ()  [unwired: 1 in, 6 out]
        n490 = Enqueue Element(queue=w1075, element=T18."UlohaEMG", error in (no error)=w1073) -> (queue out=w1074:refnum<queue>, error out=w1072:errorcluster)  [unwired: 1 in, 1 out]
        n491 = property on="SyncStopEMG" class="Bool (strict)"("Visible"=FALSE) -> ()  [unwired: 2 in, 2 out]
        n492 = Enqueue Element(queue=w1074, element=enum16{"Wait", "Exit", "Measure"}."Wait", error in (no error)=w1072) -> (queue out=w1080:refnum<queue>, error out=w1078:errorcluster)  [unwired: 1 in, 1 out]
        n493 = property on="SyncStopEMG" class="Bool (strict)"(error in=w1078, "Val(Sgnl)"=TRUE ("Value (Signaling)")) -> (error out=w1077:errorcluster)  [unwired: 1 in, 1 out]
      }
      event "StopMeasureACC": Value Change {
        n494 = event-data() -> ()  [unwired: 1 in, 6 out]
        n495 = Enqueue Element(queue=w1086, element=T7."UlohaACC", error in (no error)=w1084) -> (queue out=w1085:refnum<queue>, error out=w1083:errorcluster)  [unwired: 1 in, 1 out]
        n496 = property on="SyncStopACC" class="Bool (strict)"("Visible"=FALSE) -> ()  [unwired: 2 in, 2 out]
        n497 = Enqueue Element(queue=w1085, element=enum16{"Wait", "Exit", "Measure"}."Wait", error in (no error)=w1083) -> (queue out=w1091:refnum<queue>, error out=w1089:errorcluster)  [unwired: 1 in, 1 out]
        n498 = property on="SyncStopACC" class="Bool (strict)"(error in=w1089, "Val(Sgnl)"=TRUE ("Value (Signaling)")) -> (error out=w1088:errorcluster)  [unwired: 1 in, 1 out]
      }
      event "StopMeasureEEG": Value Change {
        n499 = event-data() -> ()  [unwired: 1 in, 6 out]
        n500 = Enqueue Element(queue=w1097, element=T7."UlohaEEG", error in (no error)=w1095) -> (queue out=w1096:refnum<queue>, error out=w1094:errorcluster)  [unwired: 1 in, 1 out]
        n501 = property on="SyncStopEEG" class="Bool (strict)"("Visible"=FALSE) -> ()  [unwired: 2 in, 2 out]
        n502 = Enqueue Element(queue=w1096, element=enum16{"Wait", "Exit", "Measure"}."Wait", error in (no error)=w1094) -> (queue out=w1102:refnum<queue>, error out=w1100:errorcluster)  [unwired: 1 in, 1 out]
        n503 = property on="SyncStopEEG" class="Bool (strict)"(error in=w1100, "Val(Sgnl)"=TRUE ("Value (Signaling)")) -> (error out=w1099:errorcluster)  [unwired: 1 in, 1 out]
      }
      event "StopMeasureEKG": Value Change {
        n504 = event-data() -> ()  [unwired: 1 in, 6 out]
        n505 = Enqueue Element(queue=w1113, element=T21."UlohaEKG", error in (no error)=w1112) -> (queue out=w1110:refnum<queue>, error out=w1108:errorcluster)  [unwired: 1 in, 1 out]
        n506 = Enqueue Element(queue=w1110, element=T21."Wait", error in (no error)=w1108) -> (queue out=w1109:refnum<queue>, error out=w1106:errorcluster)  [unwired: 1 in, 1 out]
        n507 = property on="SyncStopEKG" class="Bool (strict)"(error in=w1106, "Value"=TRUE ("SyncStop 2")) -> (error out=w1105:errorcluster)  [unwired: 1 in, 1 out]
      }
      event "GraphEKG": Scale Range Change {
        n508 = event-data() -> ("NewRange"=w1118:T39)  [unwired: 1 in, 7 out]
        n509 = Unbundle By Name(w1118) -> ("Minimum"=w1114:dbl, "Maximum"=w1115:dbl)
        n510 = property on="EKGHRV" class="XYGraph (strict)"("XScale.Maximum"=w1115, "XScale.Minimum"=w1114) -> ()  [unwired: 2 in, 2 out]
      }
      event "GraphEEG3": Scale Range Change {
        n511 = event-data() -> ("NewRange"=w1123:T39)  [unwired: 1 in, 7 out]
        n512 = Unbundle By Name(w1123) -> ("Minimum"=w1120:dbl, "Maximum"=w1119:dbl)
        n513 = property on="GraphEEG4" class="WFGraph (strict)"("XScale.Maximum"=w1119, "XScale.Minimum"=w1120) -> ()  [unwired: 2 in, 2 out]
      }
      event "DeleteSignalEKG": Value Change {
        n514 = event-data() -> ()  [unwired: 1 in, 6 out]
        n515 = Enqueue Element(queue=w1131, element=T22."UlohaEKG", error in (no error)=w1130) -> (queue out=w1128:refnum<queue>, error out=w1127:errorcluster)  [unwired: 1 in, 1 out]
        n516 = Enqueue Element(queue=w1128, element=T22."DeleteSignalEKG", error in (no error)=w1127) -> (queue out=w1124:refnum<queue>, error out=w1125:errorcluster)  [unwired: 1 in, 1 out]
      }
      event "DeleteSignalEMG": Value Change {
        n517 = event-data() -> ()  [unwired: 1 in, 6 out]
        n518 = Enqueue Element(queue=w1139, element=T22."UlohaEMG", error in (no error)=w1138) -> (queue out=w1136:refnum<queue>, error out=w1135:errorcluster)  [unwired: 1 in, 1 out]
        n519 = Enqueue Element(queue=w1136, element=T23."DeleteSignal", error in (no error)=w1135) -> (queue out=w1133:refnum<queue>, error out=w1134:errorcluster)  [unwired: 1 in, 1 out]
      }
      event "DeleteSignalEEG": Value Change {
        n520 = event-data() -> ()  [unwired: 1 in, 6 out]
        n521 = Enqueue Element(queue=w1147, element=T22."UlohaEEG", error in (no error)=w1146) -> (queue out=w1144:refnum<queue>, error out=w1143:errorcluster)  [unwired: 1 in, 1 out]
        n522 = Enqueue Element(queue=w1144, element=T24."DeleteSignal", error in (no error)=w1143) -> (queue out=w1141:refnum<queue>, error out=w1142:errorcluster)  [unwired: 1 in, 1 out]
      }
      event "DeleteSignalACC": Value Change {
        n523 = event-data() -> ()  [unwired: 1 in, 6 out]
        n524 = Enqueue Element(queue=w1155, element=T22."UlohaACC", error in (no error)=w1154) -> (queue out=w1152:refnum<queue>, error out=w1151:errorcluster)  [unwired: 1 in, 1 out]
        n525 = Enqueue Element(queue=w1152, element=T24."DeleteSignal", error in (no error)=w1151) -> (queue out=w1149:refnum<queue>, error out=w1150:errorcluster)  [unwired: 1 in, 1 out]
      }
      event "StartMeasureEKG": Value Change {
        n526 = event-data() -> ()  [unwired: 1 in, 6 out]
        n527 = Enqueue Element(queue=w1169, element=T21."UlohaEKG", error in (no error)=w1168) -> (queue out=w1166:refnum<queue>, error out=w1164:errorcluster)  [unwired: 1 in, 1 out]
        n528 = Enqueue Element(queue=w1166, element=T22."DeleteSignalEKG", error in (no error)=w1164) -> (queue out=w1165:refnum<queue>, error out=w1163:errorcluster)  [unwired: 1 in, 1 out]
        n529 = Enqueue Element(queue=w1165, element=T21."Measure", error in (no error)=w1163) -> (queue out=w1160:refnum<queue>, error out=w1158:errorcluster)  [unwired: 1 in, 1 out]
        n530 = Enqueue Element(queue=w1160, element=T7."Wait", error in (no error)=w1158) -> (queue out=w1159:refnum<queue>, error out=w1157:errorcluster)  [unwired: 1 in, 1 out]
      }
      event "GraphEMG": Shortcut Menu Activation? {
        n531 = event-data() -> ("MenuRef"=w1170:refnum<k9>)  [unwired: 1 in, 4 out]
        n532 = Delete Menu Items(9:w1170) -> ()  [unwired: 3 in, 2 out]
        n533 = event-data() -> ()  [unwired: 2 in, 1 out]
      }
      event "Délka časového okna (s)": Value Change {
        n534 = event-data() -> ()  [unwired: 1 in, 6 out]
        n535 = Enqueue Element(queue=w1178, element=T25."UlohaEKG", error in (no error)=w1176) -> (queue out=w1175:refnum<queue>, error out=w1174:errorcluster)  [unwired: 1 in, 1 out]
        n536 = Enqueue Element(queue=w1175, element=T25."ChangeTimeECG", error in (no error)=w1174) -> (queue out=w1173:refnum<queue>, error out=w1172:errorcluster)  [unwired: 1 in, 1 out]
      }
      event "Délka časového okna (s) EMG": Value Change {
        n537 = event-data() -> ()  [unwired: 1 in, 6 out]
        n538 = Enqueue Element(queue=w1186, element=T26."UlohaEMG", error in (no error)=w1185) -> (queue out=w1183:refnum<queue>, error out=w1181:errorcluster)  [unwired: 1 in, 1 out]
        n539 = Enqueue Element(queue=w1183, element=T26."ChangeTimeEMG", error in (no error)=w1181) -> (queue out=w1182:refnum<queue>, error out=w1180:errorcluster)  [unwired: 1 in, 1 out]
      }
      event "Časové okno všech signálů (s)": Value Change {
        n540 = event-data() -> ()  [unwired: 1 in, 6 out]
        n541 = Enqueue Element(queue=w1194, element=T26."UlohaEEG", error in (no error)=w1193) -> (queue out=w1191:refnum<queue>, error out=w1189:errorcluster)  [unwired: 1 in, 1 out]
        n542 = Enqueue Element(queue=w1191, element=T27."ChangeTimeEEG", error in (no error)=w1189) -> (queue out=w1190:refnum<queue>, error out=w1188:errorcluster)  [unwired: 1 in, 1 out]
      }
      event "SavePNGEMG": Value Change {
        n543 = event-data() -> ()  [unwired: 1 in, 6 out]
        n544 = Enqueue Element(queue=w1202, element=T26."UlohaEMG", error in (no error)=w1201) -> (queue out=w1200:refnum<queue>, error out=w1198:errorcluster)  [unwired: 1 in, 1 out]
        n545 = Enqueue Element(queue=w1200, element=T26."SavePNG", error in (no error)=w1198) -> (queue out=w1199:refnum<queue>, error out=w1197:errorcluster)  [unwired: 1 in, 1 out]
      }
      event "SavePNG": Value Change {
        n546 = event-data() -> ()  [unwired: 1 in, 6 out]
        n547 = Enqueue Element(queue=w1210, element=T28."UlohaEKG", error in (no error)=w1209) -> (queue out=w1207:refnum<queue>, error out=w1205:errorcluster)  [unwired: 1 in, 1 out]
        n548 = Enqueue Element(queue=w1207, element=T28."SavePNG", error in (no error)=w1205) -> (queue out=w1206:refnum<queue>, error out=w1204:errorcluster)  [unwired: 1 in, 1 out]
      }
      event "SavePNGACC": Value Change {
        n549 = event-data() -> ()  [unwired: 1 in, 6 out]
        n550 = Enqueue Element(queue=w1218, element=T28."UlohaACC", error in (no error)=w1217) -> (queue out=w1215:refnum<queue>, error out=w1213:errorcluster)  [unwired: 1 in, 1 out]
        n551 = Enqueue Element(queue=w1215, element=T28."SavePNG", error in (no error)=w1213) -> (queue out=w1214:refnum<queue>, error out=w1212:errorcluster)  [unwired: 1 in, 1 out]
      }
      event "SaveCSV": Value Change {
        n552 = event-data() -> ()  [unwired: 1 in, 6 out]
        n553 = Enqueue Element(queue=w1226, element=T29."UlohaEKG", error in (no error)=w1225) -> (queue out=w1223:refnum<queue>, error out=w1220:errorcluster)  [unwired: 1 in, 1 out]
        n554 = Enqueue Element(queue=w1223, element=T29."SaveCSV", error in (no error)=w1220) -> (queue out=w1222:refnum<queue>, error out=w1221:errorcluster)  [unwired: 1 in, 1 out]
      }
      event "GraphEKG": Mouse Down {
        n555 = event-data() -> ("Coords"=→"CoordsEKG":T40)  [unwired: 1 in, 7 out]
        n556 = Enqueue Element(queue=w1235, element=T27."UlohaEKG", error in (no error)=w1234) -> (queue out=w1232:refnum<queue>, error out=w1231:errorcluster)  [unwired: 1 in, 1 out]
        n557 = Enqueue Element(queue=w1232, element=T7."Cursor", error in (no error)=w1231) -> (queue out=w1230:refnum<queue>, error out=w1229:errorcluster)  [unwired: 1 in, 1 out]
        n558 = property on="EKGxHRV" class="Bool (strict)"("Value"=FALSE ("EKGxHRV")) -> ()  [unwired: 2 in, 2 out]
      }
      event "GraphACC": Mouse Down {
        n559 = event-data() -> ("Coords"=→"CoordsACC":T40)  [unwired: 1 in, 7 out]
        n560 = Enqueue Element(queue=w1244, element=T27."UlohaACC", error in (no error)=w1243) -> (queue out=w1241:refnum<queue>, error out=w1240:errorcluster)  [unwired: 1 in, 1 out]
        n561 = Enqueue Element(queue=w1241, element=T7."Cursor", error in (no error)=w1240) -> (queue out=w1239:refnum<queue>, error out=w1238:errorcluster)  [unwired: 1 in, 1 out]
      }
      event "GraphEEG3": Mouse Down {
        n562 = event-data() -> ("Coords"=→"CoordsEEGAlpha":T40)  [unwired: 1 in, 7 out]
        n563 = Enqueue Element(queue=w1254, element=T27."UlohaEEG", error in (no error)=w1253) -> (queue out=w1251:refnum<queue>, error out=w1250:errorcluster)  [unwired: 1 in, 1 out]
        n564 = Enqueue Element(queue=w1251, element=T7."Cursor", error in (no error)=w1250) -> (queue out=w1249:refnum<queue>, error out=w1248:errorcluster)  [unwired: 1 in, 1 out]
        "AlphaxBeta" <- TRUE ("AlphaxBeta")
      }
      event "GraphEEG4": Mouse Down {
        n565 = event-data() -> ("Coords"=→"CoordsEEGBeta":T40)  [unwired: 1 in, 7 out]
        n566 = Enqueue Element(queue=w1264, element=T27."UlohaEEG", error in (no error)=w1263) -> (queue out=w1261:refnum<queue>, error out=w1260:errorcluster)  [unwired: 1 in, 1 out]
        n567 = Enqueue Element(queue=w1261, element=T7."Cursor", error in (no error)=w1260) -> (queue out=w1259:refnum<queue>, error out=w1258:errorcluster)  [unwired: 1 in, 1 out]
        n568 = property on="AlphaxBeta" class="Bool (strict)"("Value"=FALSE ("AlphaxBeta")) -> ()  [unwired: 2 in, 2 out]
      }
      event "GraphEMG": Mouse Down {
        n569 = event-data() -> ("Coords"=→"CoordsEMG":T40)  [unwired: 1 in, 7 out]
        n570 = Enqueue Element(queue=w1273, element=T27."UlohaEMG", error in (no error)=w1272) -> (queue out=w1270:refnum<queue>, error out=w1269:errorcluster)  [unwired: 1 in, 1 out]
        n571 = Enqueue Element(queue=w1270, element=T7."Cursor", error in (no error)=w1269) -> (queue out=w1268:refnum<queue>, error out=w1267:errorcluster)  [unwired: 1 in, 1 out]
      }
      event "EKGHRV": Mouse Down {
        n572 = event-data() -> ("Coords"=→"CoordsHRV":T40)  [unwired: 1 in, 7 out]
        n573 = Enqueue Element(queue=w1283, element=T27."UlohaEKG", error in (no error)=w1282) -> (queue out=w1280:refnum<queue>, error out=w1279:errorcluster)  [unwired: 1 in, 1 out]
        n574 = Enqueue Element(queue=w1280, element=T7."Cursor", error in (no error)=w1279) -> (queue out=w1278:refnum<queue>, error out=w1277:errorcluster)  [unwired: 1 in, 1 out]
        "EKGxHRV" <- TRUE ("EKGxHRV")
      }
      event "SaveCSVEEG": Value Change {
        n575 = event-data() -> ()  [unwired: 1 in, 6 out]
        n576 = Enqueue Element(queue=w1292, element=T29."UlohaEEG", error in (no error)=w1291) -> (queue out=w1289:refnum<queue>, error out=w1286:errorcluster)  [unwired: 1 in, 1 out]
        n577 = Enqueue Element(queue=w1289, element=T29."SaveCSV", error in (no error)=w1286) -> (queue out=w1288:refnum<queue>, error out=w1287:errorcluster)  [unwired: 1 in, 1 out]
      }
      event "Zobrazit signál č._EEG": Value Change {
        n578 = event-data() -> ()  [unwired: 1 in, 6 out]
        n579 = Enqueue Element(queue=w1300, element=T31."UlohaEEG", error in (no error)=w1299) -> (queue out=w1297:refnum<queue>, error out=w1296:errorcluster)  [unwired: 1 in, 1 out]
        n580 = Enqueue Element(queue=w1297, element=T30."ShowGraphEEG", error in (no error)=w1296) -> (queue out=w1294:refnum<queue>, error out=w1293:errorcluster)  [unwired: 1 in, 1 out]
      }
      event "Zobrazit signál č._ACC": Value Change {
        n581 = event-data() -> ()  [unwired: 1 in, 6 out]
        n582 = Enqueue Element(queue=w1308, element=T32."UlohaACC", error in (no error)=w1307) -> (queue out=w1306:refnum<queue>, error out=w1305:errorcluster)  [unwired: 1 in, 1 out]
        n583 = Enqueue Element(queue=w1306, element=T32."ShowGraphACC", error in (no error)=w1305) -> (queue out=w1304:refnum<queue>, error out=w1303:errorcluster)  [unwired: 1 in, 1 out]
      }
      event "Délka časového okna (s) ACC": Value Change {
        n584 = event-data() -> ()  [unwired: 1 in, 6 out]
        n585 = Enqueue Element(queue=w1316, element=T32."UlohaACC", error in (no error)=w1315) -> (queue out=w1313:refnum<queue>, error out=w1311:errorcluster)  [unwired: 1 in, 1 out]
        n586 = Enqueue Element(queue=w1313, element=T32."ChangeTimeACC", error in (no error)=w1311) -> (queue out=w1312:refnum<queue>, error out=w1310:errorcluster)  [unwired: 1 in, 1 out]
      }
      event "SaveCSVEMG": Value Change {
        n587 = event-data() -> ()  [unwired: 1 in, 6 out]
        n588 = Enqueue Element(queue=w1324, element=T29."UlohaEMG", error in (no error)=w1323) -> (queue out=w1321:refnum<queue>, error out=w1318:errorcluster)  [unwired: 1 in, 1 out]
        n589 = Enqueue Element(queue=w1321, element=T29."SaveCSV", error in (no error)=w1318) -> (queue out=w1320:refnum<queue>, error out=w1319:errorcluster)  [unwired: 1 in, 1 out]
      }
      event "SaveCSVACC": Value Change {
        n590 = event-data() -> ()  [unwired: 1 in, 6 out]
        n591 = Enqueue Element(queue=w1332, element=T29."UlohaACC", error in (no error)=w1331) -> (queue out=w1329:refnum<queue>, error out=w1326:errorcluster)  [unwired: 1 in, 1 out]
        n592 = Enqueue Element(queue=w1329, element=T29."SaveCSV", error in (no error)=w1326) -> (queue out=w1328:refnum<queue>, error out=w1327:errorcluster)  [unwired: 1 in, 1 out]
      }
      event "StartMeasureEMG": Value Change {
        n593 = event-data() -> ()  [unwired: 1 in, 6 out]
        n594 = Enqueue Element(queue=w1343, element=T21."UlohaEMG", error in (no error)=w1342) -> (queue out=w1337:refnum<queue>, error out=w1335:errorcluster)  [unwired: 1 in, 1 out]
        n595 = Enqueue Element(queue=w1337, element=T23."DeleteSignal", error in (no error)=w1335) -> (queue out=w1336:refnum<queue>, error out=w1334:errorcluster)  [unwired: 1 in, 1 out]
        n596 = Enqueue Element(queue=w1336, element=T21."Measure", error in (no error)=w1334) -> (queue out=w1341:refnum<queue>, error out=w1340:errorcluster)  [unwired: 1 in, 1 out]
      }
      event "Zobrazit signál č.": Value Change {
        n597 = event-data() -> ()  [unwired: 1 in, 6 out]
        n598 = Enqueue Element(queue=w1351, element=T26."UlohaEMG", error in (no error)=w1350) -> (queue out=w1345:refnum<queue>, error out=w1344:errorcluster)  [unwired: 1 in, 1 out]
        n599 = Enqueue Element(queue=w1345, element=T31."ShowGraphEMG", error in (no error)=w1344) -> (queue out=w1348:refnum<queue>, error out=w1347:errorcluster)  [unwired: 1 in, 1 out]
      }
      event "StartMeasureEEG": Value Change {
        n600 = event-data() -> ()  [unwired: 1 in, 6 out]
        n601 = Enqueue Element(queue=w1362, element=T21."UlohaEEG", error in (no error)=w1361) -> (queue out=w1357:refnum<queue>, error out=w1355:errorcluster)  [unwired: 1 in, 1 out]
        n602 = Enqueue Element(queue=w1357, element=T24."DeleteSignal", error in (no error)=w1355) -> (queue out=w1356:refnum<queue>, error out=w1354:errorcluster)  [unwired: 1 in, 1 out]
        n603 = Enqueue Element(queue=w1356, element=T24."Measure", error in (no error)=w1354) -> (queue out=w1360:refnum<queue>, error out=w1359:errorcluster)  [unwired: 1 in, 1 out]
      }
      event "Zobrazit graf č.": Value Change {
        n604 = event-data() -> ()  [unwired: 1 in, 6 out]
        n605 = Enqueue Element(queue=w1370, element=T33."UlohaEKG", error in (no error)=w1369) -> (queue out=w1368:refnum<queue>, error out=w1366:errorcluster)  [unwired: 1 in, 1 out]
        n606 = Enqueue Element(queue=w1368, element=T33."ShowGraphECG", error in (no error)=w1366) -> (queue out=w1367:refnum<queue>, error out=w1365:errorcluster)  [unwired: 1 in, 1 out]
      }
      event "StartMeasure": Value Change {
        n607 = event-data() -> ()  [unwired: 1 in, 6 out]
        n608 = Enqueue Element(queue=w1375, element=T18."PlaygroundMeas", error in (no error)=w1373) -> (queue out=w1374:refnum<queue>, error out=w1372:errorcluster)  [unwired: 1 in, 1 out]
        n609 = Enqueue Element(queue=w1374, element=enum16{"Wait", "Exit", "Measure"}."Measure", error in (no error)=w1372) -> (queue out=w1378:refnum<queue>, error out=w1377:errorcluster)  [unwired: 1 in, 1 out]
      }
      event "DeleteSignal": Value Change {
        n610 = event-data() -> ()  [unwired: 1 in, 6 out]
        n611 = Enqueue Element(queue=w1386, element=T21."PlaygroundMeas", error in (no error)=w1385) -> (queue out=w1383:refnum<queue>, error out=w1381:errorcluster)  [unwired: 1 in, 1 out]
        n612 = Enqueue Element(queue=w1383, element=T21."DeleteSignal", error in (no error)=w1381) -> (queue out=w1382:refnum<queue>, error out=w1380:errorcluster)  [unwired: 1 in, 1 out]
      }
      event "SendToFilter": Value Change {
        n613 = event-data() -> ()  [unwired: 1 in, 6 out]
        n614 = Enqueue Element(queue=w1394, element=T34."PlaygroundFiltr", error in (no error)=w1393) -> (queue out=w1391:refnum<queue>, error out=w1389:errorcluster)  [unwired: 1 in, 1 out]
        n615 = Enqueue Element(queue=w1391, element=T34."Wait", error in (no error)=w1389) -> (queue out=w1390:refnum<queue>, error out=w1388:errorcluster)  [unwired: 1 in, 1 out]
      }
      event "SaveFileButton": Value Change {
        n616 = event-data() -> ()  [unwired: 1 in, 6 out]
        n617 = Enqueue Element(queue=w1399, element=T35."SaveFile", error in (no error)=w1398) -> (queue out=w1397:refnum<queue>, error out=w1396:errorcluster)  [unwired: 1 in, 1 out]
      }
      event "Filtr": Value Change {
        n618 = event-data() -> ()  [unwired: 1 in, 6 out]
        n619 = Enqueue Element(queue=w1407, element=T36."PlaygroundFiltr", error in (no error)=w1404) -> (queue out=w1406:refnum<queue>, error out=w1403:errorcluster)  [unwired: 1 in, 1 out]
        n620 = Enqueue Element(queue=w1406, element=T36."FilterSignal", error in (no error)=w1403) -> (queue out=w1405:refnum<queue>, error out=w1402:errorcluster)  [unwired: 1 in, 1 out]
      }
      event "HintEKG": Value Change {
        n621 = event-data() -> ()  [unwired: 1 in, 6 out]
        n622 = Enqueue Element(queue=w1415, element=T16."UlohaEKG", error in (no error)=w1412) -> (queue out=w1414:refnum<queue>, error out=w1411:errorcluster)  [unwired: 1 in, 1 out]
        n623 = Enqueue Element(queue=w1414, element=T16."HintEKG", error in (no error)=w1411) -> (queue out=w1413:refnum<queue>, error out=w1410:errorcluster)  [unwired: 1 in, 1 out]
      }
      event "HintEMG": Value Change {
        n624 = event-data() -> ()  [unwired: 1 in, 6 out]
        n625 = Enqueue Element(queue=w1423, element=T16."UlohaEMG", error in (no error)=w1420) -> (queue out=w1422:refnum<queue>, error out=w1419:errorcluster)  [unwired: 1 in, 1 out]
        n626 = Enqueue Element(queue=w1422, element=T37."HintEMG", error in (no error)=w1419) -> (queue out=w1421:refnum<queue>, error out=w1418:errorcluster)  [unwired: 1 in, 1 out]
      }
      event "HintEEG": Value Change {
        n627 = event-data() -> ()  [unwired: 1 in, 6 out]
        n628 = Enqueue Element(queue=w1431, element=T16."UlohaEEG", error in (no error)=w1428) -> (queue out=w1430:refnum<queue>, error out=w1427:errorcluster)  [unwired: 1 in, 1 out]
        n629 = Enqueue Element(queue=w1430, element=T38."HintEEG", error in (no error)=w1427) -> (queue out=w1429:refnum<queue>, error out=w1426:errorcluster)  [unwired: 1 in, 1 out]
      }
      event "HintACC": Value Change {
        n630 = event-data() -> ()  [unwired: 1 in, 6 out]
        n631 = Enqueue Element(queue=w1439, element=T16."UlohaACC", error in (no error)=w1436) -> (queue out=w1438:refnum<queue>, error out=w1435:errorcluster)  [unwired: 1 in, 1 out]
        n632 = Enqueue Element(queue=w1438, element=T32."HintACC", error in (no error)=w1435) -> (queue out=w1437:refnum<queue>, error out=w1434:errorcluster)  [unwired: 1 in, 1 out]
      }
    }
    n633 = Wait Until Next ms Multiple(millisecond multiple=u32 250) -> ()  [unwired: 1 out]
  }
  n634 = Release Queue(queue=w16, error in (no error)=w15) -> (error out=w12:errorcluster)  [unwired: 1 in, 2 out]
  n635 = Unregister For Events(event registration refnum=w13, error in=w12) -> (error out=w11:errorcluster)
  n636 = Destroy User Event(user event=w10, error in=w11) -> ()  [unwired: 1 out]
